vi "G#Debugger_GUI.vi"() -> ()   [LabVIEW 2020, in "G#Debugger.lvlib"]
doc: "Debugger for G# Objects."
uses:
  <vilib>/addons/_AddQ/G#Debugger/G#Debugger.lvlib
  <vilib>/addons/_AddQ/G#Object/G#Object.lvclass
  <vilib>/addons/_AddQ/G#Debugger/private/G#Debugger_DebugDialog.vi
  <vilib>/Platform/browser.llb/Open URL in Default Browser (string).vi
  <vilib>/addons/_AddQ/G#Debugger/G#Debugger_CloneUI.vi
panel:
  in  "OpClnUI":bool
  in  "RootClass":i32(ring) caption="G# Clone"
  in  "AggregatorsTags":i32(listbox)
  in  "Help":bool
  out "Application Instance":string
  in  "Window Behaviour":bool
  in  "Window Transparency":u8(slide) max=75 scale=0.0..75.0
  in  "External Create Process Running":bool
  in  "Tab Control":enum32{"Objects", "Trace", "Active Debug"}(tab)
  in  "Aggregators":i32(listbox)
  in  "AggregatesTags":i32(listbox)
  in  "Sorting":enum16{"Creation order", "By aggregation"}(ring)
  in  "Aggregates":i32(listbox)
  in  "Highlight Aggregates?":bool=TRUE
  out "To String":string
  in  "Attributes":bool
  in  "Inheritance":i32(listbox)
  in  "Destroy":bool
  in  "Object Tree":string(tree)
  in  "Refresh":bool
  out "# of Users":i32
  out "Counter":bool
  out "Ref Valid":bool
  out "Object Name":string
  out "Full Class Name":string
  in  "Poll Time (ms)":i32=200 min=0
  in  "Garbage collect":bool
  out "Object ID":u32 format="%x"
  in  "Hide Empty Classes?":bool=TRUE
  out "Owner":string
  in  "ShowAggregators":bool
  in  "Filter Expression":string
  in  "Trace Direction":bool=TRUE
  in  "Clear":bool
  in  "Save":bool
  out "Trace":string
  in  "Max Lines":u32=1000
  out "Run State":string
  out "CachedObjId":u32 caption="Object ID" format="%x"
  in  "Abort VI":bool
  in  "Run VI":bool
  in  "Open Panel":bool
  in  "DebugTree":string(tree)
  in  "Enable Active Debug":bool
  out "Icon":picture
  out "Cached Ref Valid":bool
  in  "Wait Until Done":bool=TRUE
  out "Cached Reference Class Name":string
  out "G# Version":string
  # "G# Debugger"
  # "These logs will also always appear in the NI LabVIEW Desktop Execution Trace, even without debugger running."
  # "The last created reference is automatically cashed and copied to all the new selected , opened or executed methods 'reference in'."
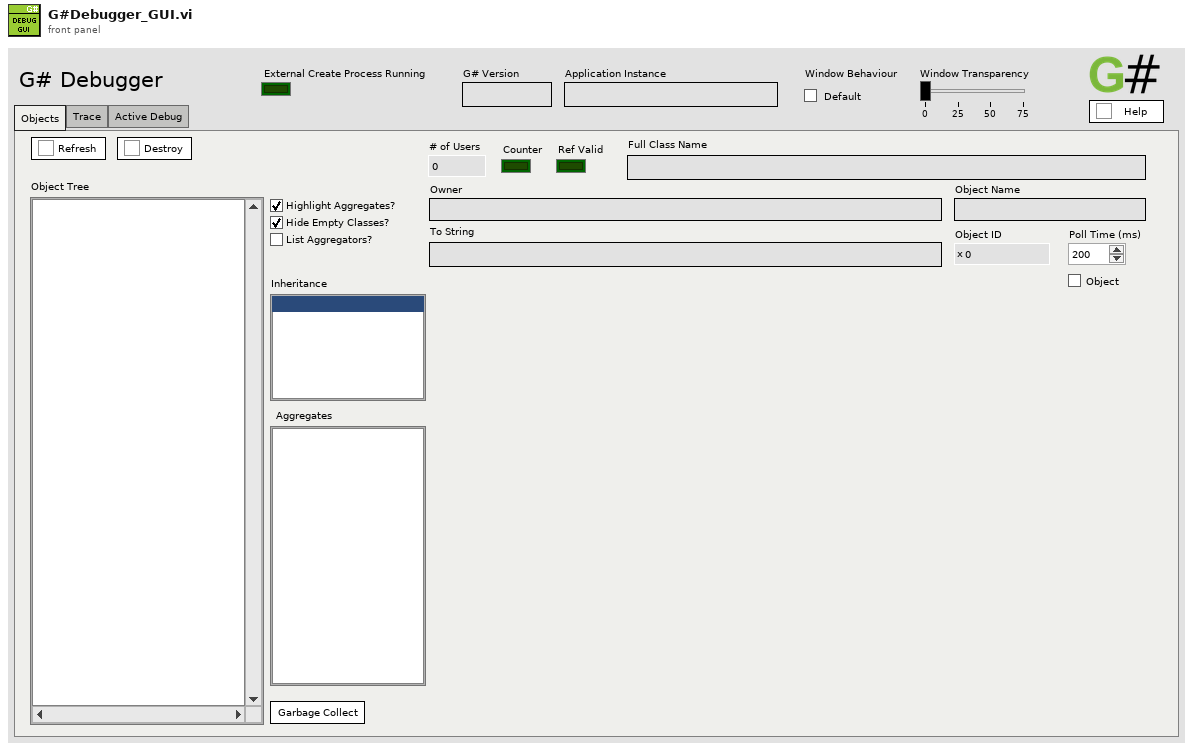
[diagram p1: front panel]
types:
  T1 = typedef "G#Debugger.lvlib/G#Debugger_Refs.ctl" = cluster{"class information dvr":refnum<data-value>, "sub panel dvr":refnum<data-value>, "GUI event":refnum<user-event>, "Active Project":refnum<vi>, "Front Panel":refnum<vi>}
  T2 = enum8{"Enabled", "Disabled", "Disabled and Grayed Out"}
  T3 = cluster{"Active Item Row Number":i32, "name":string}
  T4 = enum32{"Invalid", "Default", "Floating", "Floating/Auto-Hide", "Modal"}
  T5 = typedef "G#Debugger.lvlib/G#Debugger_SubPanelInfo.ctl" = cluster{"Ref":refnum<class "G#Object.lvclass">, "class hierarchy":T6[], "class attributes":path[], "object attributes":path[], "inheritance index":i32, "is class attributes":bool, "vi reference":refnum<vi>}
  T6 = typedef "G#Object.lvclass/G#Object_ClassHierarchy.ctl" = cluster{"ClassName":string, "FullClassName":string, "ClassPath":path, "IsLeaf":bool}
  T7 = enum32{"Bad", "Idle", "Run top level", "Running"}
  T8 = cluster{"Active Item Row Number":i32, "name":string}[]
  T9 = typedef "imagedata.ctl" = cluster{"image type":i32, "image depth":i32, "image":u8[], "mask":u8[], "colors":u32[], "Rectangle":cluster{"left":i16, "top":i16, "right":i16, "bottom":i16}}
  T10 = typedef "G#Object.lvclass/G#Object_EventType.ctl" = enum16{"Created new", "Looked up existing", "Deleted", "Forced delete", "Not deleted", "Garbage collected", "Cleared", "User", "Error", "External create object", "External create class attributes", "Created class attributes", "Run constructor", "Run constructor done", "Run open method", "Run open method done"}
  T11 = typedef "G#Object.lvclass/G#Object_ObjectInfoType.ctl" = cluster{"ObjectName":string, "ObjectID":u32, "Users":i32, "Counter":bool, "AttributeRefs":u32[], "FullClassName":string, "ClassName":string, "CreateMethod":T12, "GenericDestructorExists":bool, "Owner":string}
  T12 = typedef "G#Object.lvclass/G#Object_CreateMethod.ctl" = enum16{"Create", "Create or look up existing", "Look up existing"}
  T13 = typedef "G#Debugger.lvlib/G#Debugger_TreeElement.ctl" = cluster{"Name":string, "Tag":string, "ParentTag":string, "Position":i32}
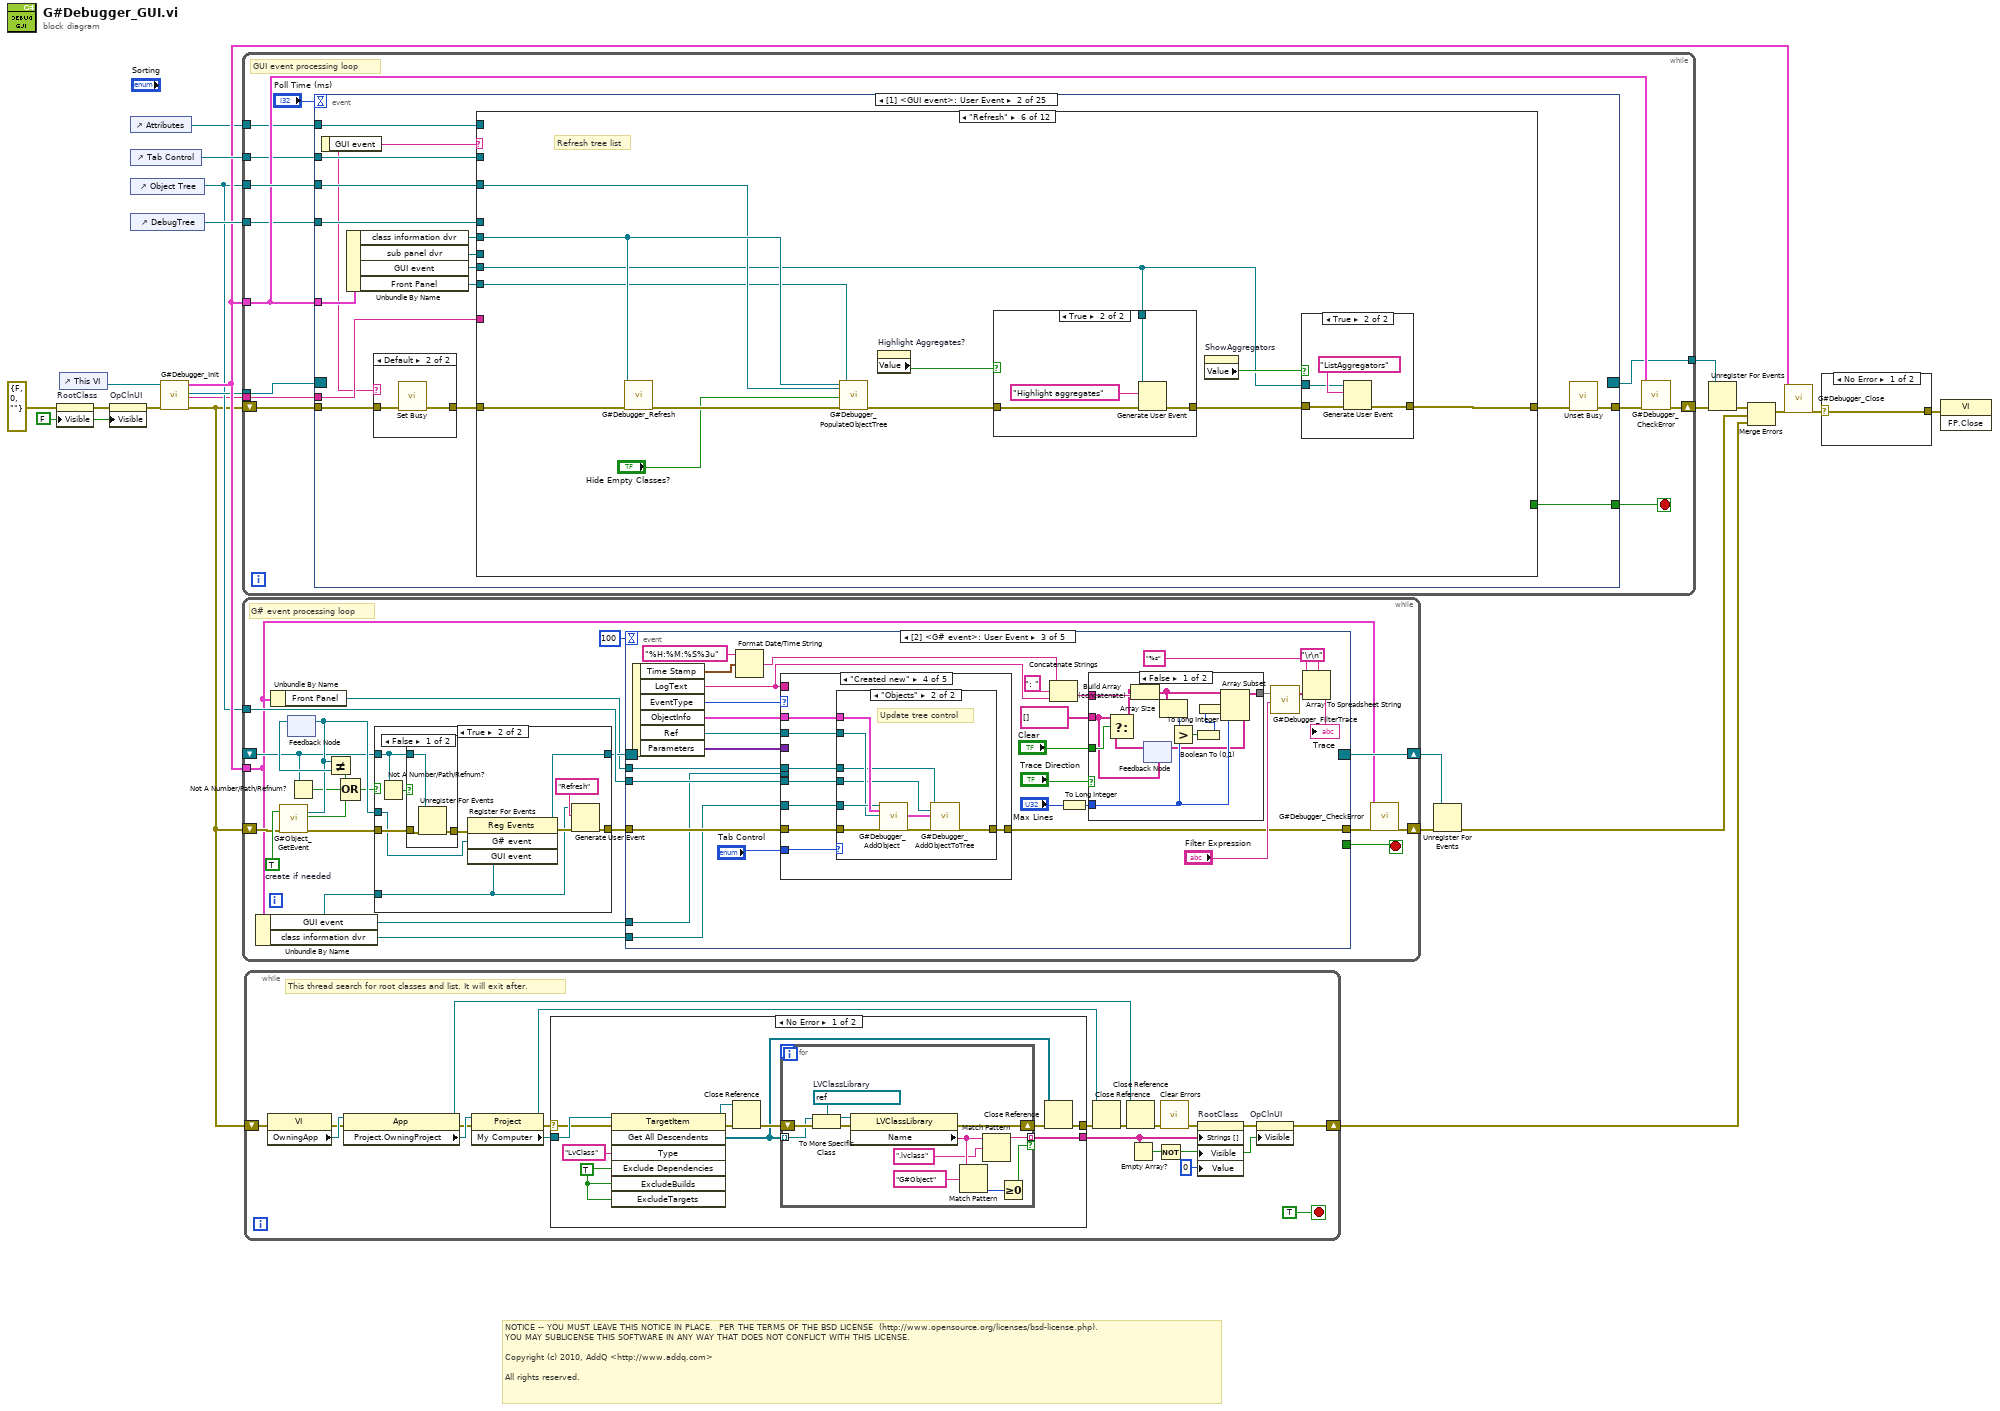
[diagram p0: block diagram]
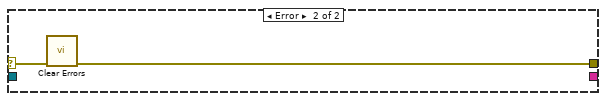
[diagram p2: hidden frame]
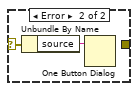
[diagram p3: hidden frame]
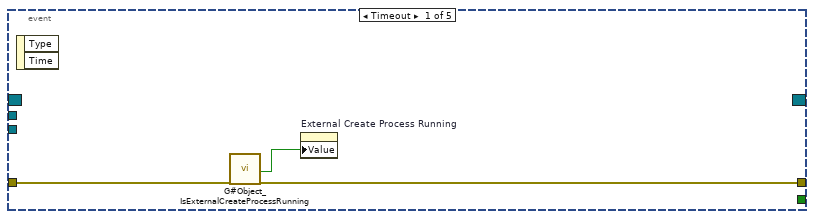
[diagram p6: hidden frame]
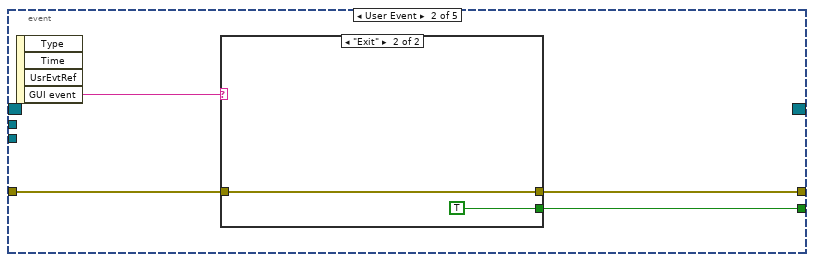
[diagram p7: hidden frame]
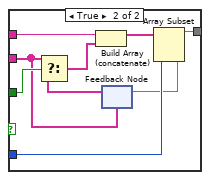
[diagram p9: hidden frame]
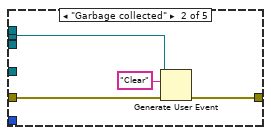
[diagram p11: hidden frame]
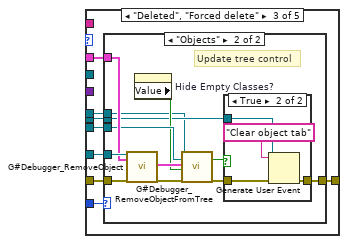
[diagram p12: hidden frame]
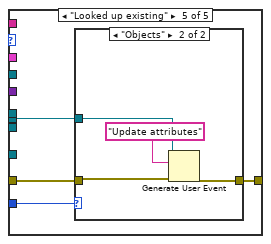
[diagram p16: hidden frame]
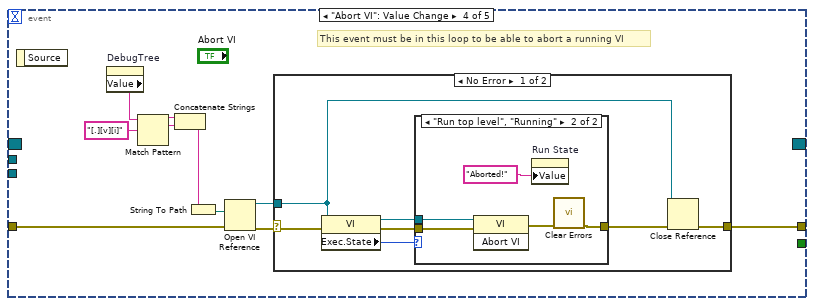
[diagram p18: hidden frame]
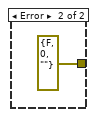
[diagram p20: hidden frame]
diagram:
  w4 = FALSE ("Visible")
  # "NOTICE -- YOU MUST LEAVE THIS NOTICE IN PLACE.  PER THE TERMS OF THE BSD LICENSE  (http://www.opensource.org/licenses/bsd-license.php).\nYOU MAY SUBLICENSE THIS SOFTWARE IN ANY WAY THAT DOES NOT CONFLICT WITH THIS LICENSE.\n\nCopyright (c) 2010, AddQ <http://www.addq.com>\n\nAll rights reserved."
  n1 = property on="RootClass" class="Ring (strict)"(error in=errorcluster {"status"=FALSE, "code"=0, "source"=""} ("error in (no error)"), "Visible"=w4) -> (error out=w3:errorcluster)  [unwired: 1 in, 1 out]
  n2 = control-ref of="This VI"() -> (w10:refnum<vi>)
  n3 = property on="OpClnUI" class="Bool"(error in=w3, "Visible"=w4) -> (error out=w1:errorcluster)  [unwired: 1 in, 1 out]
  n4 = control-ref of="Tab Control"() -> (w23:refnum<vi>)
  n5 = control-ref of="Attributes"() -> (w9:refnum<vi>)
  n6 = control-ref of="Object Tree"() -> (w12:refnum<vi>)
  n7 = control-ref of="DebugTree"() -> (w22:refnum<vi>)
  n8 = call <vilib>:"G#Debugger_Init.vi"("This VI"=w10, "error in (no error)"=w1) -> ("refs"=w21:T1, "GUI Event Registration Refnum"=w19:refnum<event-registration>, "Application Instance"=w11:string, "error out"=w6:errorcluster)  [unwired: 14 in]
  n9 = while {
    shift-right: [w34] -> w18
    shift-left: w6 -> [w29]
    tunnel: w12 -> [w36]
    tunnel: w21 -> [w32]
    tunnel: w23 -> [w31]
    tunnel: w22 -> [w30]
    tunnel: w19 -> [w28]
    tunnel: [w25] -> w17
    tunnel: w11 -> [w26]
    tunnel: w9 -> [w24]
    stop <- w35 stop-if-true
    # "GUI event processing loop"
    n10 = event shown="[1] <GUI event>: User Event" {
      selector: w28 -> [_ _ _ _ _ _ _ _ _ _ _ _ _ _ _ _ _ _ _ _ _ _ _ _ _]
      dyn-events: [_ _ _ _ _ _ _ _ _ _ _ _ _ _ _ _ _ _ _ _ _ _ _ _ _] -> w25
      timeout: "Poll Time (ms)" -> [_ _ _ _ _ _ _ _ _ _ _ _ _ _ _ _ _ _ _ _ _ _ _ _ _]
      tunnel: w29 -> [w42 w76 w473 w480 w490 w504 w508 w550 w585 w606 w613 w617 w624 w629 w632 w654 w679 w687 w727 w734 w737 w744 w759 w764 w794]
      tunnel: [w39 w78 w473 w480 w489 w503 w507 w532 w584 w605 w614 w615 w622 w626 w636 w649 w676 w686 w726 w733 w736 w744 w758 w761 w779] -> w33
      tunnel: w36 -> [_ w89 w474 w481 _ _ _ w549 _ _ w612 _ _ _ _ w648 _ _ _ _ _ _ _ w763 _]
      tunnel: [_ w88 _ _ _ FALSE _ _ _ _ _ _ _ _ _ _ _ _ _ _ _ _ _ _ _] -> w35
      tunnel: w32 -> [w46 w87 _ _ w488 w502 w506 w545 _ w604 _ w616 w623 _ w634 w645 _ w685 _ _ _ _ _ w760 _]
      tunnel: w31 -> [_ w84 _ _ _ _ _ _ _ _ _ _ _ _ _ _ _ _ _ _ _ _ _ _ _]
      tunnel: w30 -> [_ w82 _ _ _ _ _ _ _ _ _ _ _ _ _ _ _ w688 _ _ _ _ _ _ _]
      tunnel: w26 -> [_ w81 _ _ _ _ _ _ _ _ _ _ _ _ _ _ _ w684 _ _ _ _ _ _ _]
      tunnel: w24 -> [_ w74 _ _ _ _ _ _ _ _ _ _ _ _ _ _ _ _ _ _ _ _ _ _ _]
      event Timeout {
        # "redraw FP"
        n11 = event-data() -> ()  [unwired: 1 in, 2 out]
        n12 = Unbundle By Name(w46) -> ("Front Panel"=w40:refnum<vi>, "GUI event"=w45:refnum<user-event>)
        n13 = property on="Tab Control" class="TabCtl (strict)"(error in=w42) -> (error out=w43:errorcluster, "Value"=w44:enum32{"Objects", "Trace", "Active Debug"})  [unwired: 1 in, 1 out]
        n14 = case shown="Default" w44 {
          tunnel: w43 -> [w47 w57 w71]
          tunnel: w45 -> [_ w53 _]
          tunnel: [w47 w54 w70] -> w41
          frame Default {
          }
          frame "Objects" {
            # "Check for dead objects, every\n5th timeout."
            n15 = Generate User Event(user event=w53, event data cluster="Update attributes" ("event data"), error in=w57) -> (error out=w55:errorcluster)  [unwired: 1 in, 1 out]
            n16 = feedback #1(u64 0) -> (w49:u64)
            n17 = Quotient & Remainder(x=w49, y=u64 5) -> (x-y*floor(x/y)=w52:u64)  [unwired: 1 out]
            n18 = Increment(x=w49) -> (x+1=w48:u64)
            n19 = feedback-in #1(w48) -> ()
            n20 = case shown="0" w52 {
              tunnel: w55 -> [w58 w63]
              tunnel: [w58 w62] -> w54
              tunnel: w53 -> [_ w61]
              frame Default {
              }
              frame 0 {
                n21 = call <vilib>:"G#Object_CleanUp.vi"("error in (no error)"=w63) -> ("any dead objects?"=w59:bool, "error out"=w60:errorcluster)  [unwired: 17 in]
                n22 = case shown="True" w59 {
                  tunnel: w60 -> [w64 w67]
                  tunnel: [w64 w66] -> w62
                  tunnel: w61 -> [_ w65]
                  frame False {
                  }
                  frame True {
                    # "Object died, refresh"
                    n23 = Generate User Event(user event=w65, event data cluster="Refresh" ("event data"), error in=w67) -> (error out=w66:errorcluster)  [unwired: 1 in, 1 out]
                  }
                }
              }
            }
          }
          frame "Active Debug" {
            w73 = FALSE  # set
            n24 = call <vilib>:"G#Debugger_CachedObject.vi"("error in (no error)"=w71, "set"=w73) -> ("not a refnum?"=w72:bool, "error out"=w70:errorcluster)  [unwired: 15 in, 1 out]
            n25 = Not(x=w72) -> (.not. x?=w69:bool)
            n26 = property on="Cached Ref Valid" class="Bool (strict)"("Value"=w69) -> ()  [unwired: 2 in, 2 out]
          }
        }
        n27 = property class="Pnl"(reference=w40, error in=w41, "DeferPanUpdts"=FALSE ("Defer Panel Updates"), "DeferPanUpdts"=TRUE ("Defer Panel Updates")) -> (error out=w39:errorcluster)  [unwired: 1 out]
      }
      event User Event {
        n28 = event-data() -> ("GUI event"=w77:string)  [unwired: 1 in]
        n29 = Unbundle By Name(w87) -> ("class information dvr"=w86:refnum<data-value>, "sub panel dvr"=w85:refnum<data-value>, "GUI event"=w83:refnum<user-event>, "Front Panel"=w80:refnum<vi>)
        n30 = case shown="Default" w77 {
          tunnel: w76 -> [w90 w92]
          tunnel: [w90 w91] -> w75
          frame "Clear object tab", "Update attributes" {
          }
          frame Default {
            n31 = call <vilib>:"Set Busy.vi"("error in (no error)"=w92) -> ("error out"=w91:errorcluster)  [unwired: 9 in, 1 out]
          }
        }
        n32 = case shown="\"Refresh\"" w77 {
          selector: w77 -> [_ _ _ _ _ _ _ _ _ w320 _ _]
          tunnel: [w93 w94 w128 w138 w145 w151 w175 w184 w276 w316 w326 w370] -> w79
          tunnel: w75 -> [w93 w123 w129 w138 w144 w161 w179 w181 w277 w316 w331 w375]
          tunnel: [_ _ _ _ TRUE _ _ _ _ _ _ _] -> w88
          tunnel: w86 -> [_ _ _ _ _ w159 w177 w187 _ _ w329 w373]
          tunnel: w89 -> [_ w116 _ _ _ w158 w178 _ _ _ w325 w369]
          tunnel: w85 -> [_ _ _ _ _ _ _ w186 _ _ _ _]
          tunnel: w84 -> [_ w124 _ _ _ _ _ _ _ _ _ _]
          tunnel: w83 -> [_ w121 w127 _ _ w150 w174 w185 _ _ _ _]
          tunnel: w82 -> [_ w117 _ _ _ _ _ _ _ _ _ _]
          tunnel: w81 -> [_ w112 _ _ _ _ _ _ _ _ _ _]
          tunnel: w80 -> [_ w98 _ _ _ w154 w172 _ _ _ w321 w365]
          tunnel: w74 -> [_ _ _ _ _ _ _ w182 _ _ _ _]
          frame Default {
          }
          frame "Init" {
            w95 = FALSE ("ShowAggregators")
            w99 = TRUE ("Highlight Aggregates?")
            n33 = call <vilib>:"G#Object_GetRootClassVersion.vi"("error in (no error)"=w123) -> ("version"=→"G# Version":string, "error out"=w105:errorcluster)  [unwired: 17 in]
            n34 = invoke on="Method VI Panel" class="SubPanel" method="Remove VI"(error in=w105) -> (error out=w104:errorcluster)  [unwired: 2 in, 2 out]
            n35 = call <vilib>:"G#Debugger_ClearTree.vi"("Front Panel"=w98, "Tree"=w116, "error in (no error)"=w104) -> ("error out"=w114:errorcluster)  [unwired: 16 in]
            n36 = Equal?(x=w112, y="Main Application Instance") -> (x = y?=w110:bool)
            n37 = call <vilib>:"G#Object_IsExternalCreateProcessRunning.vi"("error in (no error)"=w114) -> ("external create process running?"=w106:bool, "error out"=w113:errorcluster)  [unwired: 15 in, 2 out]
            n38 = Select(t=T2."Disabled and Grayed Out" ("Disabled"), s=w110, f=T2."Enabled" ("Disabled")) -> (s? t:f=w107:T2)
            n39 = property on="External Create Process Running" class="Bool (strict)"("Value"=w106) -> ()  [unwired: 2 in, 2 out]
            n40 = property class="TabCtl (strict)"(reference=w124, error in=w113, "Value"=enum32{"Objects", "Trace", "Active Debug"}."Objects") -> (error out=w120:errorcluster)  [unwired: 1 out]
            n41 = property on="Aggregators" class="LstBox (strict)"("Visible"=FALSE) -> ()  [unwired: 2 in, 2 out]
            n42 = property on="Enable Active Debug" class="Bool (strict)"(error in=w120, "Value"=FALSE ("Enable Active Debug"), "DisabledEnum"=w107) -> (error out=w103:errorcluster)  [unwired: 1 in, 1 out]
            n43 = property on="Aggregates" class="LstBox (strict)"("Number of Rows"=u32 16) -> ()  [unwired: 2 in, 2 out]
            n44 = call <vilib>:"G#Debugger_ClearTree.vi"("Front Panel"=w98, "Tree"=w117, "error in (no error)"=w103) -> ("error out"=w115:errorcluster)  [unwired: 16 in]
            n45 = Generate User Event(user event=w121, event data cluster="Clear controls" ("event data"), error in=w115) -> (user event out=w102:refnum<user-event>, error out=w101:errorcluster)  [unwired: 1 in]
            n46 = property on="Hide Empty Classes?" class="Bool (strict)"("Value"=w99) -> ()  [unwired: 2 in, 2 out]
            n47 = property on="Highlight Aggregates?" class="Bool (strict)"("Value"=w99) -> ()  [unwired: 2 in, 2 out]
            n48 = Generate User Event(user event=w102, event data cluster="Refresh" ("event data"), error in=w101) -> (error out=w94:errorcluster)  [unwired: 1 in, 1 out]
            n49 = property on="ShowAggregators" class="Bool (strict)"("Value"=w95) -> ()  [unwired: 2 in, 2 out]
            n50 = property on="RootClass" class="Ring (strict)"("Visible"=w95) -> ()  [unwired: 2 in, 2 out]
            n51 = property on="OpClnUI" class="Bool"("Visible"=w95) -> ()  [unwired: 2 in, 2 out]
            "Application Instance" <- w112
          }
          frame "Clear controls" {
            w130 = ""
            n52 = property on="Run State" class="Str"("Value"=w130) -> ()  [unwired: 2 in, 2 out]
            n53 = property on="Cached Reference Class Name" class="Str"("Value"=w130) -> ()  [unwired: 2 in, 2 out]
            n54 = call "Empty Picture"() -> ("empty picture"=w132:picture)
            n55 = property on="Cached Ref Valid" class="Bool (strict)"("Value"=FALSE ("Counter")) -> ()  [unwired: 2 in, 2 out]
            n56 = property on="Icon" class="Pict"("Value"=w132) -> ()  [unwired: 2 in, 2 out]
            n57 = property on="Trace" class="Str"("Value"=w130) -> ()  [unwired: 2 in, 2 out]
            n58 = property on="CachedObjId" class="DigNum (strict)"("Value"=u32 0 ("Object ID")) -> ()  [unwired: 2 in, 2 out]
            n59 = Generate User Event(user event=w127, event data cluster="Clear object tab" ("event data"), error in=w129) -> (error out=w128:errorcluster)  [unwired: 1 in, 1 out]
          }
          frame "Clear object tab" {
            w134 = 0 ("Top Row")
            w135 = string[] [] ("Item Names")
            w136 = -1 ("Inheritance")
            w137 = ""
            w141 = FALSE ("Counter")
            n60 = property on="Object Name" class="Str"("Value"=w137) -> ()  [unwired: 2 in, 2 out]
            n61 = property on="To String" class="Str"("Value"=w137) -> ()  [unwired: 2 in, 2 out]
            n62 = property on="Full Class Name" class="Str"("Value"=w137) -> ()  [unwired: 2 in, 2 out]
            n63 = property on="Owner" class="Str"("Value"=w137) -> ()  [unwired: 2 in, 2 out]
            n64 = property on="Counter" class="Bool (strict)"("Value"=w141) -> ()  [unwired: 2 in, 2 out]
            n65 = property on="Ref Valid" class="Bool (strict)"("Value"=w141) -> ()  [unwired: 2 in, 2 out]
            n66 = property on="# of Users" class="DigNum (strict)"("Value"=0 ("Nr of Users")) -> ()  [unwired: 2 in, 2 out]
            n67 = property on="Object ID" class="DigNum (strict)"("Value"=u32 0 ("Object ID")) -> ()  [unwired: 2 in, 2 out]
            n68 = property on="Aggregates" class="LstBox (strict)"("Value"=w136, "Item Names"=w135, "Top Row"=w134) -> ()  [unwired: 2 in, 2 out]
            n69 = property on="Inheritance" class="LstBox (strict)"("Value"=w136, "Item Names"=w135, "Top Row"=w134) -> ()  [unwired: 2 in, 2 out]
            n70 = property on="Aggregators" class="LstBox (strict)"("Value"=w136, "Item Names"=w135, "Top Row"=w134) -> ()  [unwired: 2 in, 2 out]
          }
          frame "Exit" {
            n71 = property on="Enable Active Debug" class="Bool (strict)"(error in=w144) -> (error out=w143:errorcluster, "Value"=w142:bool)  [unwired: 1 in, 1 out]
            n72 = case shown="True" w142 {
              tunnel: [w147 w149] -> w145
              tunnel: w143 -> [w147 w148]
              frame False {
              }
              frame True {
                n73 = call <vilib>:"GarbageCollector.vi"("error in (no error)"=w148) -> ("error out"=w149:errorcluster)  [unwired: 16 in, 2 out]
              }
            }
          }
          frame "Refresh" {
            # "Refresh tree list"
            n74 = call <vilib>:"G#Debugger_Refresh.vi"("Objects dvr"=w159, "error in (no error)"=w161) -> ("error out"=w160:errorcluster)  [unwired: 17 in]
            n75 = call <vilib>:"G#Debugger_PopulateObjectTree.vi"("Objects dvr"=w159, "Tree"=w158, "hide empty classes?"="Hide Empty Classes?", "error in (no error)"=w160, "Front Panel"=w154) -> ("error out"=w156:errorcluster)  [unwired: 14 in]
            n76 = property on="Highlight Aggregates?" class="Bool (strict)"() -> ("Value"=w155:bool)  [unwired: 2 in, 2 out]
            n77 = case shown="True" w155 {
              tunnel: [w167 w170] -> w152
              tunnel: w156 -> [w167 w169]
              tunnel: w150 -> [_ w168]
              frame False {
              }
              frame True {
                n78 = Generate User Event(user event=w168, event data cluster="Highlight aggregates" ("event data"), error in=w169) -> (error out=w170:errorcluster)  [unwired: 1 in, 1 out]
              }
            }
            n79 = property on="ShowAggregators" class="Bool (strict)"() -> ("Value"=w153:bool)  [unwired: 2 in, 2 out]
            n80 = case shown="True" w153 {
              tunnel: w152 -> [w162 w165]
              tunnel: [w162 w164] -> w151
              tunnel: w150 -> [_ w163]
              frame False {
              }
              frame True {
                n81 = Generate User Event(user event=w163, event data cluster="ListAggregators" ("event data"), error in=w165) -> (error out=w164:errorcluster)  [unwired: 1 in, 1 out]
              }
            }
          }
          frame "Clear" {
            # "Clears tree and object cache"
            n82 = call <vilib>:"G#Debugger_ClearTree.vi"("Front Panel"=w172, "Tree"=w178, "error in (no error)"=w179) -> ("error out"=w180:errorcluster)  [unwired: 16 in]
            n83 = call <vilib>:"G#Debugger_Clear.vi"("Objects dvr"=w177, "error in (no error)"=w180) -> ("error out"=w176:errorcluster)  [unwired: 17 in]
            n84 = Generate User Event(user event=w174, event data cluster="Clear object tab" ("event data"), error in=w176) -> (error out=w175:errorcluster)  [unwired: 1 in, 1 out]
          }
          frame "Update attributes" {
            n85 = Empty String/Path?(string/path="Object Tree") -> (empty?=w189:bool)
            n86 = case shown="False" w189 {
              tunnel: w181 -> [w207 w261]
              tunnel: w187 -> [w206 _]
              tunnel: w186 -> [w205 w259]
              tunnel: "Object Tree" -> [w204 _]
              tunnel: "Attributes" -> [w192 _]
              tunnel: "Inheritance" -> [w203 _]
              tunnel: [w200 w255] -> w183
              tunnel: w185 -> [w195 w254]
              tunnel: w182 -> [w193 _]
              frame False {
                # "An item is selected"
                n87 = call <vilib>:"G#Debugger_UpdateAttributes.vi"("Objects dvr"=w206, "Subpanel dvr"=w205, "tag"=w204, "class attributes"=w192, "inheritance index"=w203, "error in (no error)"=w207) -> ("string"=w196:string, "Only read attributes"=w199:bool, "attributes reference"=w198:refnum<vi>, "attributes value"=w197:variant, "valid object"=w202:bool, "# of users?"=w194:i32, "error out"=w201:errorcluster)  [unwired: 7 in]
                n88 = case shown="True" w202 {
                  tunnel: w201 -> [w215 w235]
                  tunnel: [w209 w236] -> w200
                  tunnel: w199 -> [_ w225]
                  tunnel: w198 -> [_ w221]
                  tunnel: w197 -> [_ w228]
                  tunnel: w196 -> [_ w238]
                  tunnel: w195 -> [w208 _]
                  tunnel: w194 -> [_ w237]
                  tunnel: w193 -> [_ w234]
                  tunnel: w192 -> [_ w231]
                  frame False {
                    # "Subpanel info is invalid->Clear"
                    n89 = invoke on="Attributes" class="SubPanel" method="Remove VI"(error in=w215) -> (error out=w214:errorcluster)  [unwired: 2 in, 2 out]
                    n90 = call <vilib>:"G#Object_CleanUp.vi"("error in (no error)"=w214) -> ("any dead objects?"=w212:bool, "error out"=w213:errorcluster)  [unwired: 17 in]
                    n91 = case shown="True" w212 {
                      tunnel: [w217 w219] -> w210
                      tunnel: w213 -> [w217 w219]
                      tunnel: ["Clear object tab" ("event data") "Refresh" ("event data")] -> w211
                      frame False {
                      }
                      frame True {
                      }
                    }
                    n92 = Generate User Event(user event=w208, event data cluster=w211, error in=w210) -> (error out=w209:errorcluster)  [unwired: 1 in, 1 out]
                  }
                  frame True {
                    # "Valid item"
                    n93 = case shown="False" w225 {
                      tunnel: w235 -> [w251 w252]
                      tunnel: w234 -> [w248 _]
                      tunnel: [w250 w252] -> w226
                      tunnel: w221 -> [w249 _]
                      tunnel: w231 -> [w247 _]
                      frame False {
                        n94 = call <vilib>:"G#Debugger_ShowAttributes.vi"("VIRef"=w249, "SubPanel"=w248, "ClassAttributes"=w247, "error in (no error)"=w251) -> ("error out"=w250:errorcluster)  [unwired: 14 in, 1 out]
                      }
                      frame True {
                      }
                    }
                    n95 = property on="# of Users" class="DigNum (strict)"("Value"=w237) -> ()  [unwired: 2 in, 2 out]
                    n96 = Select(t="class attributes" ("y"), s=w231, f="attributes" ("y")) -> (s? t:f=w230:string)
                    n97 = Not(x=w225) -> (.not. x?=w224:bool)
                    n98 = invoke class="VI" method="Ctrl Val.Get"(reference=w221, error in=w226, "Control Name"=w230) -> (reference out=w220:refnum<vi>, error out=w227:errorcluster, "Get Control Value Variant"=w229:variant)  [unwired: 1 in, 1 out]
                    n99 = Not Equal?(x=w229, y=w228) -> (x != y?=w223:bool)
                    n100 = Or(x=w224, y=w223) -> (x .or. y?=w222:bool)
                    n101 = case shown="True" w222 {
                      tunnel: [w239 w245] -> w236
                      tunnel: w227 -> [w239 w243]
                      tunnel: w220 -> [_ w242]
                      tunnel: w230 -> [_ w241]
                      tunnel: w228 -> [_ w240]
                      frame False {
                      }
                      frame True {
                        n102 = invoke class="VI" method="Ctrl Val.Set"(reference=w242, error in=w243, "Control Name"=w241, "Value"=w240) -> (error out=w246:errorcluster)  [unwired: 1 in, 4 out]
                        n103 = property on="Attributes" class="SubPnl"(error in=w246, "DisabledEnum"=T2."Enabled" ("Disabled")) -> (error out=w245:errorcluster)  [unwired: 1 in, 1 out]
                      }
                    }
                    "To String" <- w238
                  }
                }
              }
              frame True {
                # "No item selected in tree"
                n104 = invoke on="Attributes" class="SubPanel" method="Remove VI"(error in=w261) -> (error out=w260:errorcluster)  [unwired: 2 in, 2 out]
                n105 = in-place {
                  in-place-border: w260 -> [w266]
                  in-place-border: [w264] -> w257
                  # "Force a subpanel update!"
                  n106 = in-place-dvr #2(w259) -> (w265:T5)  [unwired: 1 out]
                  n107 = Unbundle By Name(w265) -> ("vi reference"=w262:refnum<vi>)
                  n108 = Not A Number/Path/Refnum?(number/path/refnum=w262) -> (NaN/Path/Refnum?=w263:bool)
                  n109 = case shown="False" w263 {
                    tunnel: w266 -> [w269 w270]
                    tunnel: [w268 w270] -> w264
                    tunnel: w262 -> [w267 _]
                    frame False {
                      n110 = Close Reference(reference=w267, error in (no error)=w269) -> (error out=w268:errorcluster)
                    }
                    frame True {
                    }
                  }
                  n111 = in-place-dvr #2(w265) -> (w258:errorcluster)  [unwired: 1 out]
                }
                n112 = Merge Errors(w258, w257) -> (w256:errorcluster)
                n113 = Generate User Event(user event=w254, event data cluster="Clear object tab" ("event data"), error in=w256) -> (error out=w255:errorcluster)  [unwired: 1 in, 1 out]
              }
            }
            n114 = call <vilib>:"Clear Errors.vi"("error in (no error)"=w183) -> ("error out"=w184:errorcluster)  [unwired: 5 in, 1 out]
          }
          frame "Run VI" {
            n115 = property on="DebugTree" class="Tree (strict)"() -> ("Value"=w271:string)  [unwired: 2 in, 2 out]
            n116 = Match Pattern(string=w271, regular expression="[.][v][i]") -> (before substring=w274:string, match substring=w273:string)  [unwired: 1 in, 2 out]
            n117 = Concatenate Strings(w274, w273) -> (w272:string)
            n118 = String To Path(string=w272) -> (path=w278:path)
            n119 = Open VI Reference(vi path=w278, error in (no error)=w277) -> (vi reference=w280:refnum<vi>, error out=w279:errorcluster)  [unwired: 4 in]
            n120 = case shown="No Error" w279 {
              selector: w279 -> [w285 _]
              tunnel: [w291 errorcluster {"status"=FALSE, "code"=0, "source"=""} ("error in (no error)")] -> w276
              tunnel: w280 -> [w284 _]
              tunnel: w278 -> [w289 _]
              frame No Error {
                n121 = stacked-sequence {
                  tunnel: w289 -> [w297]
                  tunnel: [w297] -> w288
                  frame #0 {
                    "Run State" <- "Running..." ("Run State")
                  }
                }
                n122 = property class="VI"(reference=w284, error in=w285) -> (error out=w282:errorcluster, "Exec.State"=w283:T7, "Exec.IsReentrant"=w286:bool)  [unwired: 1 out]
                n123 = case shown="Default" w283 {
                  tunnel: [FALSE TRUE w294 w295] -> w287
                  tunnel: w286 -> [_ _ w294 w295]
                  frame Default {
                  }
                  frame "Idle" {
                  }
                  frame "Run top level" {
                  }
                  frame "Running" {
                  }
                }
                n124 = case shown="True" w287 {
                  tunnel: [w303 w311] -> w290
                  tunnel: w282 -> [w303 w306]
                  tunnel: w288 -> [w302 _]
                  tunnel: [w299 w314] -> w281
                  tunnel: w283 -> [w298 _]
                  tunnel: w284 -> [_ w307]
                  frame False {
                    n125 = Strip Path(path=w302) -> (name=w301:string)  [unwired: 1 out]
                    n126 = Format Into String(format string="%s is not reentrant or in idle execution state! (%s)", w301, w298) -> (resulting string=w299:string)  [unwired: 2 in, 1 out]
                  }
                  frame True {
                    n127 = call <vilib>:"G#Debugger_RunVI.vi"("vi reference"=w307, "wait until done"="Wait Until Done", "error in (no error)"=w306) -> ("class name"=→"Cached Reference Class Name":string, "object ID"=→"CachedObjId":u32, "message"=w310:string, "not a refnum?"=w305:bool, "error out"=w311:errorcluster)  [unwired: 12 in]
                    n128 = Not(x=w305) -> (.not. x?=→"Cached Ref Valid":bool)
                    n129 = Select(t=w310, s="Wait Until Done", f="Run state is not available!") -> (s? t:f=w314:string)
                  }
                }
                n130 = Close Reference(reference=w284, error in (no error)=w290) -> (error out=w291:errorcluster)
                n131 = property on="Run State" class="Str"("Value"=w281) -> ()  [unwired: 2 in, 2 out]
              }
              frame Error {
              }
            }
          }
          frame "Wait".."Wb" {
            n132 = Decimal String To Number(string=w320, offset=5, default (0L)=u32 0 ("default (0 I32)")) -> (number=w317:u32)  [unwired: 1 out]
            n133 = Wait (ms)(milliseconds to wait=w317) -> ()  [unwired: 1 out]
          }
          frame "Highlight aggregates" {
            n134 = property on="Property Node" class="Tree (strict)"(reference=w325, error in=w331) -> (error out=w330:errorcluster, "Value"=w328:string)  [unwired: 1 out]
            n135 = call <vilib>:"G#Debugger_GetObjectFromTag.vi"("Objects dvr"=w329, "Tag"=w328, "class attributes"=FALSE, "error in (no error)"=w330) -> ("Ref"=w324:refnum<class "G#Object.lvclass">, "Found"=w322:bool, "error out"=w323:errorcluster)  [unwired: 13 in]
            n136 = case shown="True" w322 {
              tunnel: [w332 w340] -> w326
              tunnel: w325 -> [_ w352]
              tunnel: w324 -> [_ w351]
              tunnel: w323 -> [w332 w349]
              tunnel: w321 -> [_ w339]
              frame False {
              }
              frame True {
                w346 = TRUE  # remove duplicates
                # "redraw FP"
                n137 = property on="Attributes" class="Bool (strict)"(error in=w349) -> (error out=w348:errorcluster, "Value"=w347:bool)  [unwired: 1 in, 1 out]
                n138 = call <vilib>:"G#Object_GetAggregatedObjects.vi"("reference in"=w351, "class attributes (F)"=w347, "remove duplicates (F)"=w346, "error in (no error)"=w348) -> ("aggregated objects"=w345:refnum<class "G#Object.lvclass">[], "error out"=w344:errorcluster)  [unwired: 12 in, 2 out]
                n139 = for {
                  tunnel: w345 -> [w355] mode=indexing
                  shift-right: [w356] -> w350
                  shift-left: w344 -> [w358]
                  tunnel: [w357] -> w333 mode=indexing if=w353
                  n140 = call-dynamic "NotARefNum.vi"("reference in"=w355) -> ("not a refnum?"=w354:bool)  [unwired: 1 in, 1 out]
                  n141 = case shown="False" w354 {
                    tunnel: w355 -> [w363 _]
                    tunnel: w358 -> [w362 w364]
                    tunnel: [w360 _] -> w357
                    tunnel: [w359 w364] -> w356
                    frame False {
                      # "ObjectIDs are the\ntags in the object tree"
                      n142 = call-dynamic "GetObjectID.vi"("reference in"=w363, "error in (no error)"=w362) -> ("object ID"=w361:u32, "error out"=w359:errorcluster)  [unwired: 15 in, 1 out]
                      n143 = Number To Decimal String(number=w361) -> (decimal integer string=w360:string)  [unwired: 1 in]
                    }
                    frame True {
                    }
                  }
                  n144 = Not(x=w354) -> (.not. x?=w353:bool)
                }
                n145 = control-ref of="Aggregates"() -> (w338:refnum<vi>)
                n146 = control-ref of="AggregatesTags"() -> (w337:refnum<vi>)
                n147 = Array Size(array=w333) -> (size(s)=w336:i32)
                n148 = call <vilib>:"G#Debugger_Highlight.vi"("Tree"=w352, "Aggregates"=w338, "ObjectIDs"=w333, "error in (no error)"=w350, "AggregatesTags"=w337) -> ("error out"=w341:errorcluster)  [unwired: 14 in]
                n149 = Greater Or Equal?(x=w336, y=8) -> (x >= y?=w335:bool)
                n150 = property class="Pnl"(reference=w339, error in=w341, "DeferPanUpdts"=FALSE ("Defer Panel Updates"), "DeferPanUpdts"=TRUE ("Defer Panel Updates")) -> (error out=w340:errorcluster)  [unwired: 1 out]
                n151 = property on="Aggregates" class="LstBox (strict)"("Scrollbar Visible"=w335) -> ()  [unwired: 2 in, 2 out]
              }
            }
          }
          frame "ListAggregators" {
            n152 = property on="Property Node" class="Tree (strict)"(reference=w369, error in=w375) -> (error out=w374:errorcluster, "Value"=w372:string)  [unwired: 1 out]
            n153 = call <vilib>:"G#Debugger_GetObjectFromTag.vi"("Objects dvr"=w373, "Tag"=w372, "class attributes"=FALSE, "error in (no error)"=w374) -> ("Ref"=w368:refnum<class "G#Object.lvclass">, "Found"=w366:bool, "error out"=w367:errorcluster)  [unwired: 13 in]
            n154 = case shown="True" w366 {
              tunnel: [w376 w396] -> w370
              tunnel: w369 -> [_ _]
              tunnel: w368 -> [_ w395]
              tunnel: w367 -> [w376 w401]
              tunnel: w365 -> [_ w381]
              frame False {
              }
              frame True {
                # "redraw FP"
                n155 = call-dynamic "GetObjectID.vi"("reference in"=w395) -> ("object ID"=w378:u32)  [unwired: 16 in, 2 out]
                n156 = property on="Attributes" class="Bool (strict)"(error in=w401) -> (error out=w400:errorcluster, "Value"=w399:bool)  [unwired: 1 in, 1 out]
                n157 = Equal To 0?(x=w378) -> (x = 0?=w377:bool)
                n158 = case shown="False" w377 {
                  tunnel: w400 -> [w413 w464]
                  tunnel: w399 -> [w412 _]
                  tunnel: w378 -> [w406 _]
                  tunnel: [w405 w464] -> w394
                  tunnel: [w403 _] -> w387
                  tunnel: [w402 _] -> w385
                  frame False {
                    w411 = TRUE  # remove duplicates
                    n159 = call <vilib>:"G#Object_GetAllObjects.vi"("only refs (F)"=TRUE) -> ("all refs"=w408:refnum<class "G#Object.lvclass">[])  [unwired: 15 in, 3 out]
                    n160 = for {
                      tunnel: w412 -> [w420]
                      tunnel: w411 -> [w419]
                      tunnel: [w417] -> w410 mode=indexing if=w414
                      shift-right: [w418] -> w409
                      shift-left: w413 -> [w421]
                      tunnel: w408 -> [w416] mode=indexing
                      tunnel: [w416] -> w404 mode=indexing if=w414
                      n161 = call-dynamic "NotARefNum.vi"("reference in"=w416) -> ("not a refnum?"=w415:bool)  [unwired: 1 in, 1 out]
                      n162 = Not(x=w415) -> (.not. x?=w414:bool)
                      n163 = case shown="False" w415 {
                        tunnel: w421 -> [w428 w433]
                        tunnel: w420 -> [w427 _]
                        tunnel: w419 -> [w426 _]
                        tunnel: [w425 w433] -> w418
                        tunnel: w416 -> [w424 _]
                        tunnel: [w422 _] -> w417
                        frame False {
                          n164 = call <vilib>:"G#Object_GetAggregatedObjects.vi"("reference in"=w424, "class attributes (F)"=w427, "remove duplicates (F)"=w426, "error in (no error)"=w428) -> ("aggregated objects"=w423:refnum<class "G#Object.lvclass">[], "error out"=w425:errorcluster)  [unwired: 12 in, 2 out]
                          n165 = for {
                            tunnel: w423 -> [w432] mode=indexing
                            tunnel: [w431] -> w422 mode=indexing if=w429
                            n166 = call-dynamic "NotARefNum.vi"("reference in"=w432) -> ("not a refnum?"=w430:bool, "reference out"=w431:refnum<class "G#Object.lvclass">)  [unwired: 1 in]
                            n167 = Not(x=w430) -> (.not. x?=w429:bool)
                          }
                        }
                        frame True {
                        }
                      }
                    }
                    n168 = for {
                      tunnel: w410 -> [w444] mode=indexing
                      shift-right: [w440] -> w405
                      shift-left: w409 -> [w443]
                      tunnel: [w436] -> w403 mode=indexing if=w434
                      tunnel: w406 -> [w442]
                      tunnel: w404 -> [w439] mode=indexing
                      tunnel: [w435] -> w402 mode=indexing if=w434
                      # "ObjectIDs are the\ntags in the object tree"
                      n169 = for {
                        tunnel: w444 -> [w455] mode=indexing
                        tunnel: w442 -> [w453]
                        tunnel: [w450] -> w434
                        shift-right: [w451] -> w441
                        shift-left: w443 -> [w454]
                        stop <- w450 stop-if-true
                        n170 = call-dynamic "GetObjectID.vi"("reference in"=w455, "error in (no error)"=w454) -> ("object ID"=w452:u32, "error out"=w451:errorcluster)  [unwired: 15 in, 1 out]
                        n171 = Equal?(x=w453, y=w452) -> (x = y?=w450:bool)
                      }
                      n172 = case shown="True" w434 {
                        tunnel: w441 -> [w456 w463]
                        tunnel: [w456 w462] -> w440
                        tunnel: w439 -> [_ w458]
                        tunnel: [_ w460] -> w438
                        tunnel: [_ w459] -> w437
                        tunnel: [_ w457] -> w435
                        frame False {
                        }
                        frame True {
                          n173 = call-dynamic "GetObjectID.vi"("reference in"=w458) -> ("object ID"=w457:u32)  [unwired: 16 in, 2 out]
                          n174 = call-dynamic "GetObjectStatus.vi"("reference in"=w458, "simple info (F)"=TRUE, "error in (no error)"=w463) -> ("class name"=w460:string, "object name"=w459:string, "error out"=w462:errorcluster)  [unwired: 5 in, 9 out]
                        }
                      }
                      n175 = disable-structure shown="Enabled" {
                        disable-tunnel: w438 -> [w448 _]
                        disable-tunnel: w437 -> [w447 w449]
                        disable-tunnel: [w445 w449] -> w436
                        frame Enabled {
                          n176 = Format Into String(format string="%s:%s", w448, w447) -> (resulting string=w445:string)  [unwired: 2 in, 1 out]
                        }
                        frame Disabled {
                        }
                      }
                    }
                  }
                  frame True {
                  }
                }
                n177 = for {
                  tunnel: w385 -> [w469] mode=indexing
                  tunnel: w387 -> [w470] mode=indexing
                  tunnel: [w468] -> w389 mode=indexing
                  n178 = Bundle(cluster=T3 {"Active Item Row Number"=0, "name"=""}, "Active Item Row Number"=w469, "name"=w470) -> (w468:T3)
                }
                n179 = Sort 1D Array(array=w385) -> (sorted array=w384:u32[])
                n180 = Array Size(array=w384) -> (size(s)=w392:i32)
                n181 = Greater Or Equal?(x=w392, y=7) -> (x >= y?=w391:bool)
                n182 = Number To Decimal String(number=w384) -> (decimal integer string=w382:string[])  [unwired: 1 in]
                n183 = property on="Aggregators" class="LstBox (strict)"("Scrollbar Visible"=w391) -> ()  [unwired: 2 in, 2 out]
                n184 = Sort 1D Array(array=w389) -> (sorted array=w388:T8)
                n185 = for {
                  tunnel: w388 -> [w466] mode=indexing
                  tunnel: [w465] -> w386 mode=indexing
                  n186 = Unbundle By Name(w466) -> ("name"=w465:string)
                }
                n187 = property on="Aggregators" class="LstBox (strict)"(error in=w394, "Item Names"=w386) -> (error out=w393:errorcluster)  [unwired: 1 in, 1 out]
                n188 = control-ref of="AggregatorsTags"() -> (w390:refnum<vi>)
                n189 = property on="Property Node" class="LstBox (strict)"(reference=w390, "Item Names"=w382, "Value"=-1, "Top Row"=0) -> ()  [unwired: 1 in, 2 out]
                n190 = property class="Pnl"(reference=w381, error in=w393, "DeferPanUpdts"=FALSE ("Defer Panel Updates"), "DeferPanUpdts"=TRUE ("Defer Panel Updates")) -> (error out=w396:errorcluster)  [unwired: 1 out]
              }
            }
          }
        }
        n191 = call <vilib>:"Unset Busy.vi"("error in (no error)"=w79) -> ("error out"=w78:errorcluster)  [unwired: 10 in]
      }
      event "Aggregates": Double Click {
        n192 = event-data() -> ()  [unwired: 1 in, 1 out]
        n193 = control-ref of="AggregatesTags"() -> (w472:refnum<vi>)
        n194 = control-ref of="Aggregates"() -> (w471:refnum<vi>)
        n195 = property class="LstBox (strict)"(reference=w472) -> ("Item Names"=w476:string[])  [unwired: 1 in, 2 out]
        n196 = property class="LstBox (strict)"(reference=w471) -> ("Value"=w477:i32)  [unwired: 1 in, 2 out]
        n197 = Index Array(array=w476, index=w477) -> (element=w475:string)
        n198 = property class="Tree (strict)"(reference=w474, "Val(Sgnl)"=w475) -> ()  [unwired: 1 in, 2 out]
      }
      event "Aggregators": Double Click {
        n199 = event-data() -> ()  [unwired: 1 in, 1 out]
        n200 = control-ref of="AggregatorsTags"() -> (w479:refnum<vi>)
        n201 = control-ref of="Aggregators"() -> (w478:refnum<vi>)
        n202 = property class="LstBox (strict)"(reference=w478) -> ("Value"=w484:i32)  [unwired: 1 in, 2 out]
        n203 = property class="LstBox (strict)"(reference=w479) -> ("Item Names"=w483:string[])  [unwired: 1 in, 2 out]
        n204 = Index Array(array=w483, index=w484) -> (element=w482:string)
        n205 = property class="Tree (strict)"(reference=w481, "Val(Sgnl)"=w482) -> ()  [unwired: 1 in, 2 out]
      }
      event "ShowAggregators": Value Change {
        n206 = event-data() -> ("NewVal"=w486:bool)  [unwired: 1 in]
        n207 = Unbundle By Name(w488) -> ("GUI event"=w487:refnum<user-event>)
        n208 = property on="Aggregators" class="LstBox (strict)"("Visible"=w486) -> ()  [unwired: 2 in, 2 out]
        n209 = case shown="True" w486 {
          tunnel: w490 -> [w492 w496]
          tunnel: [w492 w495] -> w489
          tunnel: w487 -> [_ w494]
          tunnel: [u32 16 ("Number of Rows") u32 7 ("Number of Rows")] -> w485
          frame False {
          }
          frame True {
            n210 = Generate User Event(user event=w494, event data cluster="ListAggregators" ("event data"), error in=w496) -> (error out=w495:errorcluster)  [unwired: 1 in, 1 out]
          }
        }
        n211 = property on="Aggregates" class="LstBox (strict)"("Number of Rows"=w485) -> ()  [unwired: 2 in, 2 out]
      }
      event Panel Close? {
        n212 = event-data() -> ()  [unwired: 1 in, 3 out]
        n213 = Unbundle By Name(w502) -> ("GUI event"=w499:refnum<user-event>)
        n214 = Generate User Event(user event=w499, event data cluster="Exit" ("event data"), error in=w504) -> (error out=w503:errorcluster)  [unwired: 1 in, 1 out]
        n215 = event-data("Discard?"=TRUE) -> ()  [unwired: 1 in, 1 out]
      }
      event "Tab Control": Value Change {
        n216 = event-data() -> ("NewVal"=w509:enum32{"Objects", "Trace", "Active Debug"})  [unwired: 1 in, 4 out]
        n217 = Unbundle By Name(w506) -> ("GUI event"=w505:refnum<user-event>)
        n218 = case shown="\"Objects\"" w509 {
          tunnel: w508 -> [w513 w516]
          tunnel: [w515 w516] -> w507
          tunnel: w505 -> [w511 _]
          frame "Objects" {
            # "Refresh tree control"
            n219 = Generate User Event(user event=w511, event data cluster="Clear object tab" ("event data"), error in=w513) -> (error out=w512:errorcluster)  [unwired: 1 in, 1 out]
            n220 = Generate User Event(user event=w511, event data cluster="Refresh" ("event data"), error in=w512) -> (error out=w515:errorcluster)  [unwired: 1 in, 1 out]
          }
          frame Default {
          }
        }
      }
      event "Object Tree": Value Change {
        w561 = TRUE  # simple info
        n221 = event-data() -> ()  [unwired: 1 in, 1 out]
        n222 = property class="Tree (strict)"(reference=w549, error in=w550) -> (error out=w531:errorcluster, "Value"=w548:string)  [unwired: 1 out]
        n223 = Unbundle By Name(w545) -> ("class information dvr"=w544:refnum<data-value>, "GUI event"=w526:refnum<user-event>)
        n224 = property on="Attributes" class="Bool (strict)"(error in=w531) -> (error out=w530:errorcluster, "Value"=w529:bool)  [unwired: 1 in, 1 out]
        n225 = call <vilib>:"G#Debugger_GetObjectFromTag.vi"("Objects dvr"=w544, "Tag"=w548, "class attributes"=w529, "error in (no error)"=w530) -> ("Ref"=w555:refnum<class "G#Object.lvclass">, "error out"=w562:errorcluster)  [unwired: 13 in, 1 out]
        n226 = call-dynamic "GetObjectStatus.vi"("reference in"=w555, "simple info (F)"=w561, "error in (no error)"=w562) -> ("full class name"=→"Full Class Name":string, "# of users?"=→"# of Users":i32, "class name"=w533:string, "reference out"=w553:refnum<class "G#Object.lvclass">, "not a refnum?"=w558:bool, "object name"=→"Object Name":string, "counter?"=→"Counter":bool, "error out"=w554:errorcluster)  [unwired: 5 in, 4 out]
        n227 = Not(x=w558) -> (.not. x?=→"Ref Valid":bool)
        n228 = property on="Cached Reference Class Name" class="Str"("Value"=w533) -> ()  [unwired: 2 in, 2 out]
        n229 = call <vilib>:"G#Object_GetClassHierarchy.vi"("reference in"=w553, "error in (no error)"=w554) -> ("reference out"=w542:refnum<class "G#Object.lvclass">, "class hierarchy"=w552:T6[], "error out"=w543:errorcluster)  [unwired: 15 in]
        n230 = call-dynamic "GetObjectID.vi"("reference in"=w542, "error in (no error)"=w543) -> ("reference out"=w538:refnum<class "G#Object.lvclass">, "object ID"=w534:u32, "error out"=w539:errorcluster)  [unwired: 15 in]
        "Object ID" <- w534
        n231 = property on="CachedObjId" class="DigNum (strict)"("Value"=w534) -> ()  [unwired: 2 in, 2 out]
        n232 = for {
          tunnel: w552 -> [w574] mode=indexing
          tunnel: [w573] -> w547 mode=indexing
          n233 = Unbundle By Name(w574) -> ("ClassName"=w573:string)
        }
        n234 = call-dynamic "G#Object_GetOwner.vi"("reference in"=w538, "error in (no error)"=w539) -> ("reference out"=w536:refnum<class "G#Object.lvclass">, "owner"=→"Owner":string, "error out"=w537:errorcluster)  [unwired: 15 in]
        n235 = call <vilib>:"G#Debugger_CachedObject.vi"("cached object"=w536, "error in (no error)"=w537, "set"=TRUE) -> ("error out"=w528:errorcluster)  [unwired: 14 in, 2 out]
        n236 = case shown="True" "Highlight Aggregates?" {
          tunnel: w528 -> [w568 w572]
          tunnel: [w568 w571] -> w527
          tunnel: w526 -> [_ w569]
          frame False {
          }
          frame True {
            n237 = Generate User Event(user event=w569, event data cluster="Highlight aggregates" ("event data"), error in=w572) -> (error out=w571:errorcluster)  [unwired: 1 in, 1 out]
          }
        }
        n238 = Array Size(array=w547) -> (size(s)=w518:i32)
        n239 = Decrement(x=w518) -> (x-1=w546:i32)
        n240 = property on="Inheritance" class="LstBox (strict)"("Item Names"=w547, "Value"=w546, "Top Row"=0) -> ()  [unwired: 2 in, 2 out]
        n241 = Generate User Event(user event=w526, event data cluster="Update attributes" ("event data"), error in=w527) -> (user event out=w522:refnum<user-event>, error out=w524:errorcluster)  [unwired: 1 in]
        n242 = Greater Or Equal?(x=w518, y=8) -> (x >= y?=w520:bool)
        n243 = case shown="True" "ShowAggregators" {
          tunnel: w524 -> [w563 w566]
          tunnel: [w563 w565] -> w523
          tunnel: w522 -> [_ w564]
          frame False {
          }
          frame True {
            n244 = Generate User Event(user event=w564, event data cluster="ListAggregators" ("event data"), error in=w566) -> (error out=w565:errorcluster)  [unwired: 1 in, 1 out]
          }
        }
        n245 = property on="Inheritance" class="LstBox (strict)"("Scrollbar Visible"=w520) -> ()  [unwired: 2 in, 2 out]
        n246 = call <vilib>:"Clear Errors.vi"("error in (no error)"=w523) -> ("error out"=w532:errorcluster)  [unwired: 5 in, 1 out]
      }
      event "DebugTree": Value Change {
        n247 = event-data() -> ("NewVal"=w579:string)  [unwired: 1 in, 4 out]
        n248 = Match Pattern(string=w579, regular expression="[.][v][i]") -> (before substring=w577:string, match substring=w576:string)  [unwired: 1 in, 2 out]
        n249 = Concatenate Strings(w577, w576) -> (w575:string)
        n250 = String To Path(string=w575) -> (path=w580:path)
        n251 = Open VI Reference(vi path=w580, error in (no error)=w585) -> (vi reference=w583:refnum<vi>, error out=w582:errorcluster)  [unwired: 4 in]
        n252 = case shown="No Error" w582 {
          selector: w582 -> [w589 _]
          tunnel: [w592 w602] -> w584
          tunnel: w583 -> [w587 _]
          tunnel: [w590 w603] -> w581
          frame No Error {
            n253 = call <vilib>:"G#Debugger_SetCachedRef.vi"("MethodVIref"=w587, "error in (no error)"=w589) -> ("error out"=w588:errorcluster)  [unwired: 17 in]
            n254 = invoke on="Method VI Panel" class="SubPanel" method="Insert VI"(error in=w588, "VI Ref"=w587) -> (error out=w586:errorcluster)  [unwired: 2 in, 3 out]
            n255 = case shown="No Error" w586 {
              selector: w586 -> [w596 _]
              tunnel: [w595 w598] -> w591
              tunnel: w587 -> [w597 _]
              tunnel: [w593 w600] -> w590
              frame No Error {
                n256 = invoke class="VI" method="VI Icon.Get as Image Data"(reference=w597, error in=w596) -> (error out=w595:errorcluster, "ImageData"=w594:T9)  [unwired: 4 in, 4 out]
                n257 = call <vilib>:"Draw Flattened Pixmap.vi"("image data"=w594) -> ("new picture"=w593:picture)  [unwired: 8 in]
              }
              frame Error {
                n258 = vi-ref "G#Debugger.lvlib:G#Debugger_DebugDialog.vi"() -> (w599:refnum<vi>)
                n259 = invoke on="Method VI Panel" class="SubPanel" method="Insert VI"("VI Ref"=w599) -> (error out=w598:errorcluster)  [unwired: 3 in, 3 out]
                n260 = call "Empty Picture"() -> ("empty picture"=w600:picture)
              }
            }
            n261 = Close Reference(reference=w587, error in (no error)=w591) -> (error out=w592:errorcluster)
          }
          frame Error {
            n262 = invoke on="Method VI Panel" class="SubPanel" method="Remove VI"(error in=errorcluster {"status"=FALSE, "code"=0, "source"=""} ("error in (no error)")) -> (error out=w602:errorcluster)  [unwired: 2 in, 2 out]
            n263 = call "Empty Picture"() -> ("empty picture"=w603:picture)
          }
        }
        "Icon" <- w581
      }
      event "Run VI": Value Change {
        # "We need to fire a new event so we don't lock up the UI event."
        n264 = event-data() -> ()  [unwired: 1 in, 5 out]
        n265 = Unbundle By Name(w604) -> ("GUI event"=w607:refnum<user-event>)
        n266 = Generate User Event(user event=w607, event data cluster="Run VI" ("event data"), error in=w606) -> (error out=w605:errorcluster)  [unwired: 1 in, 1 out]
      }
      event "Attributes": Value Change {
        n267 = event-data() -> ()  [unwired: 1 in, 5 out]
        n268 = property class="Tree (strict)"(reference=w612, error in=w613) -> (reference out=w610:refnum<vi>, error out=w611:errorcluster, "Value"=w609:string)
        n269 = property class="Tree (strict)"(reference=w610, error in=w611, "Val(Sgnl)"=w609) -> (error out=w614:errorcluster)  [unwired: 1 out]
      }
      event "Inheritance": Value Change {
        n270 = event-data() -> ()  [unwired: 1 in, 5 out]
        n271 = Unbundle By Name(w616) -> ("GUI event"=w618:refnum<user-event>)
        n272 = Generate User Event(user event=w618, event data cluster="Update attributes" ("event data"), error in=w617) -> (error out=w615:errorcluster)  [unwired: 1 in, 1 out]
      }
      event "Refresh", "Hide Empty Classes?": Value Change {
        n273 = event-data() -> ()  [unwired: 1 in, 5 out]
        n274 = Unbundle By Name(w623) -> ("GUI event"=w620:refnum<user-event>)
        n275 = Generate User Event(user event=w620, event data cluster="Refresh" ("event data"), error in=w624) -> (error out=w622:errorcluster)  [unwired: 1 in, 1 out]
      }
      event "Clear": Value Change {
        n276 = event-data() -> ()  [unwired: 1 in, 5 out]
        n277 = call <vilib>:"G#Object_SendUserEvent.vi"("text"="Debugger clearing display!" ("Text"), "error in (no error)"=w629) -> ("error out"=w627:errorcluster)  [unwired: 16 in, 1 out]
        n278 = property on="Trace" class="Str"(error in=w627, "Value"="") -> (error out=w626:errorcluster)  [unwired: 1 in, 1 out]
      }
      event "Garbage collect": Value Change {
        n279 = event-data() -> ()  [unwired: 1 in, 5 out]
        n280 = Unbundle By Name(w634) -> ("GUI event"=w633:refnum<user-event>)
        n281 = call <vilib>:"G#Object_SendUserEvent.vi"("text"="Debugger garbage collected!" ("Text"), "error in (no error)"=w632) -> ("error out"=w640:errorcluster)  [unwired: 16 in, 1 out]
        n282 = call <vilib>:"GarbageCollector.vi"("only from same owner as caller? (T)"=FALSE, "error in (no error)"=w640) -> ("error out"=w631:errorcluster)  [unwired: 15 in, 2 out]
        n283 = call <vilib>:"Clear Errors.vi"("error in (no error)"=w631) -> ("error out"=w630:errorcluster)  [unwired: 5 in, 1 out]
        n284 = property on="Enable Active Debug" class="Bool (strict)"() -> ("Value"=w639:bool)  [unwired: 2 in, 2 out]
        n285 = case shown="True" w639 {
          tunnel: w630 -> [w642 w644]
          tunnel: [w642 w643] -> w635
          frame False {
          }
          frame True {
            n286 = call <vilib>:"G#Object_StartExternalCreateProcess.vi"("error in (no error)"=w644) -> ("error out"=w643:errorcluster)  [unwired: 18 in]
          }
        }
        n287 = property on="External Create Process Running" class="Bool (strict)"("Value"=w639) -> ()  [unwired: 2 in, 2 out]
        n288 = Generate User Event(user event=w633, event data cluster="Clear" ("event data"), error in=w635) -> (error out=w636:errorcluster)  [unwired: 1 in, 1 out]
      }
      event "Destroy": Value Change {
        n289 = event-data() -> ()  [unwired: 1 in, 5 out]
        n290 = Unbundle By Name(w645) -> ("class information dvr"=w646:refnum<data-value>)
        n291 = property class="Tree (strict)"(reference=w648, error in=w654) -> (error out=w653:errorcluster, "Value"=w647:string)  [unwired: 1 out]
        n292 = call <vilib>:"G#Debugger_GetObjectFromTag.vi"("Objects dvr"=w646, "Tag"=w647, "error in (no error)"=w653) -> ("Ref"=w650:refnum<class "G#Object.lvclass">, "Found"=w651:bool, "error out"=w652:errorcluster)  [unwired: 14 in]
        n293 = case shown="True" w651 {
          tunnel: w652 -> [w655 w661]
          tunnel: w650 -> [_ w663]
          tunnel: [w655 w662] -> w649
          tunnel: w648 -> [_ w660]
          tunnel: w647 -> [_ w659]
          frame False {
          }
          frame True {
            w665 = TRUE  # Simple Info
            n294 = call <vilib>:"G#Debugger_NavigateToPreviousTreeItem.vi"("Tree"=w660, "Tag"=w659, "error in (no error)"=w661) -> ("error out"=w658:errorcluster)  [unwired: 16 in]
            n295 = call <vilib>:"G#Object_SendUserEvent.vi"("text"="Debugger killed object!" ("Text"), "error in (no error)"=w658) -> ("error out"=w657:errorcluster)  [unwired: 16 in, 1 out]
            n296 = call-dynamic "GetObjectStatus.vi"("reference in"=w663, "simple info (F)"=w665, "error in (no error)"=w657) -> ("# of users?"=w664:i32, "error out"=w666:errorcluster)  [unwired: 5 in, 10 out]
            n297 = for {
              N: w664 -> [_]
              tunnel: [w667] -> w662
              tunnel: w666 -> [w670]
              tunnel: w663 -> [w669]
              # "Loop users"
              n298 = call-dynamic "NotARefNum.vi"("reference in"=w669) -> ("not a refnum?"=w668:bool)  [unwired: 1 in, 1 out]
              n299 = case shown="False" w668 {
                tunnel: [w672 w675] -> w667
                tunnel: w670 -> [w674 w675]
                tunnel: w669 -> [w673 _]
                frame False {
                  n300 = call-dynamic "Destroy.vi"("reference in"=w673, "error in (no error)"=w674) -> ("error out"=w671:errorcluster)  [unwired: 16 in, 1 out]
                  n301 = call <vilib>:"Clear Errors.vi"("error in (no error)"=w671) -> ("error out"=w672:errorcluster)  [unwired: 5 in, 1 out]
                }
                frame True {
                }
              }
            }
          }
        }
      }
      event "Save": Value Change {
        n302 = event-data() -> ()  [unwired: 1 in, 5 out]
        n303 = property on="Trace" class="Str"() -> ("Value"=w678:string)  [unwired: 2 in, 2 out]
        n304 = Write to Text File(text=w678, error in=w679) -> (error out=w677:errorcluster)  [unwired: 2 in, 2 out]
        n305 = call <vilib>:"Clear Errors.vi"("error in (no error)"=w677) -> ("error out"=w676:errorcluster)  [unwired: 5 in, 1 out]
      }
      event "Enable Active Debug": Value Change {
        n306 = event-data() -> ("NewVal"=w680:bool)  [unwired: 1 in, 4 out]
        n307 = Select(t="Debugger enabled active debug!" ("Text"), s=w680, f="Debugger disabled active debug!" ("Text")) -> (s? t:f=w691:string)
        n308 = call <vilib>:"G#Object_SendUserEvent.vi"("text"=w691, "error in (no error)"=w687) -> ("error out"=w683:errorcluster)  [unwired: 16 in, 1 out]
        n309 = call <vilib>:"G#Object_EnableDebug.vi"("set (F)"=TRUE, "debug enable (F)"=w680, "error in (no error)"=w683) -> ("error out"=w682:errorcluster)  [unwired: 14 in, 2 out]
        n310 = case shown="False" w680 {
          tunnel: w682 -> [w702 w710]
          tunnel: [w704 w712] -> w686
          tunnel: w688 -> [w703 w711]
          tunnel: w685 -> [w693 w709]
          tunnel: w684 -> [_ w706]
          frame False {
            n311 = Unbundle By Name(w693) -> ("Front Panel"=w692:refnum<vi>)
            n312 = property on="Cached Reference Class Name" class="Str"("Value"="") -> ()  [unwired: 2 in, 2 out]
            n313 = call <vilib>:"G#Debugger_CachedObject.vi"("cached object"=refnum<class "G#Object.lvclass"> refnum, "error in (no error)"=w702, "set"=TRUE) -> ("error out"=w701:errorcluster)  [unwired: 14 in, 2 out]
            n314 = call <vilib>:"GarbageCollector.vi"("error in (no error)"=w701) -> ("error out"=w695:errorcluster)  [unwired: 16 in, 2 out]
            n315 = property on="CachedObjId" class="DigNum (strict)"("Value"=u32 0 ("CachedObjId")) -> ()  [unwired: 2 in, 2 out]
            n316 = call "Empty Picture"() -> ("empty picture"=w696:picture)
            n317 = invoke on="Method VI Panel" class="SubPanel" method="Remove VI"(error in=w695) -> (error out=w694:errorcluster)  [unwired: 2 in, 2 out]
            n318 = property on="Icon" class="Pict"("Value"=w696) -> ()  [unwired: 2 in, 2 out]
            n319 = call <vilib>:"G#Debugger_ClearTree.vi"("Front Panel"=w692, "Tree"=w703, "error in (no error)"=w694) -> ("error out"=w704:errorcluster)  [unwired: 16 in]
          }
          frame True {
            n320 = Unbundle By Name(w709) -> ("Front Panel"=w705:refnum<vi>, "Active Project"=w708:refnum<vi>)
            n321 = Not A Number/Path/Refnum?(number/path/refnum=w708) -> (NaN/Path/Refnum?=w707:bool)
            n322 = case shown="False" w707 {
              tunnel: [w718 w723] -> w712
              tunnel: w711 -> [w717 _]
              tunnel: w710 -> [w715 w723]
              tunnel: w708 -> [w714 _]
              tunnel: w706 -> [_ w722]
              tunnel: w705 -> [w713 _]
              frame False {
                n323 = call <vilib>:"G#Object_StartExternalCreateProcess.vi"("error in (no error)"=w715) -> ("error out"=w716:errorcluster)  [unwired: 18 in]
                n324 = call <vilib>:"G#Debugger_PopulateActiveDebugTree.vi"("Front Panel"=w713, "Tree"=w717, "Active Project"=w714, "error in (no error)"=w716) -> ("error out"=w718:errorcluster)  [unwired: 15 in]
              }
              frame True {
                n325 = Format Into String(format string="%s not valid anymore!", w722) -> (resulting string=w721:string)  [unwired: 2 in, 1 out]
                n326 = property on="Enable Active Debug" class="Bool (strict)"("Value"=FALSE ("Enable Active Debug")) -> ()  [unwired: 2 in, 2 out]
                n327 = One Button Dialog(message=w721) -> ()  [unwired: 1 in, 1 out]
              }
            }
          }
        }
      }
      event "Window Transparency": Value Change {
        n328 = event-data() -> ()  [unwired: 1 in, 5 out]
        n329 = control-ref of="This VI"() -> (w728:refnum<vi>)
        n330 = Not Equal To 0?(x="Window Transparency") -> (x != 0?=w724:bool)
        n331 = property class="VI"(reference=w728, error in=w727, "FP:Transparency"="Window Transparency", "FP:RunTransparently"=w724) -> (error out=w726:errorcluster)  [unwired: 1 out]
      }
      event "Window Behaviour": Value Change {
        n332 = event-data() -> ()  [unwired: 1 in, 5 out]
        n333 = Select(t=T4."Floating" ("Front Panel Window:Behavior"), s="Window Behaviour", f=T4."Default" ("Front Panel Window:Behavior")) -> (s? t:f=w729:T4)
        n334 = property class="VI"(error in=w734, "FP.Behavior"=w729) -> (error out=w733:errorcluster)  [unwired: 1 in, 1 out]
      }
      event "External Create Process Running": Value Change {
        n335 = event-data() -> ()  [unwired: 1 in, 5 out]
        n336 = case shown="False" "External Create Process Running" {
          tunnel: w737 -> [w739 w741]
          tunnel: [w738 w740] -> w736
          frame False {
            n337 = call <vilib>:"G#Object_StopExternalCreateProcess.vi"("error in (no error)"=w739) -> ("error out"=w738:errorcluster)  [unwired: 17 in, 1 out]
          }
          frame True {
            n338 = call <vilib>:"G#Object_StartExternalCreateProcess.vi"("error in (no error)"=w741) -> ("error out"=w740:errorcluster)  [unwired: 18 in]
          }
        }
      }
      event "Help": Value Change {
        n339 = event-data() -> ()  [unwired: 1 in, 5 out]
        n340 = property class="App"() -> ("OS.Name"=w742:string, "OS.Version"=w743:string)  [unwired: 2 in, 2 out]
        n341 = case shown="\"Windows\"..\"Windowt\"" w742 {
          tunnel: w743 -> [_ _]
          frame Default {
            n342 = call-poly <vilib>:"Open URL in Default Browser.vi"("URL"="http://www.addq.se/document/GsharpOnlineManual.htm" ("message")) -> ()  [unwired: 5 in, 2 out]
          }
          frame "Windows".."Windowt" {
            w753 = TRUE  # run minimized? (F)
            w754 = FALSE  # wait until completion? (T)
            n343 = VI Library() -> (path=w752:path)
            n344 = Strip Path(path=w752) -> (stripped path=w751:path)  [unwired: 1 out]
            n345 = Build Path(base path=w751, name or relative path="help") -> (appended path=w749:path)
            n346 = Build Path(base path=w749, name or relative path="_AddQ") -> (appended path=w747:path)
            n347 = call <vilib>:"System Exec.vi"("run minimized? (F)"=w753, "wait until completion? (T)"=w754, "working directory"=w747, "command line"="cmd /c hh.exe \"Gsharp.chm::GsharpDebugger.htm\"") -> ()  [unwired: 4 in, 4 out]
          }
        }
      }
      event "Filter Expression": Value Change {
        n348 = event-data() -> ("NewVal"=w756:string)  [unwired: 1 in, 4 out]
        n349 = Format Into String(format string="Changed filter expression to '%s'!" ("text"), w756) -> (resulting string=w755:string)  [unwired: 2 in, 1 out]
        n350 = call <vilib>:"G#Object_SendUserEvent.vi"("text"=w755, "error in (no error)"=w759) -> ("error out"=w758:errorcluster)  [unwired: 16 in, 1 out]
      }
      event "Highlight Aggregates?": Value Change {
        n351 = event-data() -> ("NewVal"=w762:bool)  [unwired: 1 in, 4 out]
        n352 = case shown="False" w762 {
          tunnel: w764 -> [w772 w775]
          tunnel: w763 -> [w771 _]
          tunnel: [w767 w776] -> w761
          tunnel: w760 -> [w766 w774]
          frame False {
            # "redraw FP"
            n353 = call <vilib>:"G#Debugger_Highlight.vi"("Tree"=w771, "error in (no error)"=w772) -> ("error out"=w768:errorcluster)  [unwired: 17 in]
            n354 = Unbundle By Name(w766) -> ("Front Panel"=w765:refnum<vi>)
            n355 = property class="Pnl"(reference=w765, error in=w768, "DeferPanUpdts"=FALSE ("Defer Panel Updates"), "DeferPanUpdts"=TRUE ("Defer Panel Updates")) -> (error out=w767:errorcluster)  [unwired: 1 out]
          }
          frame True {
            n356 = Unbundle By Name(w774) -> ("GUI event"=w773:refnum<user-event>)
            n357 = Generate User Event(user event=w773, event data cluster="Highlight aggregates" ("event data"), error in=w775) -> (error out=w776:errorcluster)  [unwired: 1 in, 1 out]
          }
        }
      }
      event "OpClnUI": Value Change {
        n358 = event-data() -> ()  [unwired: 1 in, 1 out]
        n359 = property on="RootClass" class="Ring (strict)"(error in=w794) -> (error out=w782:errorcluster, "Strings []"=w793:string[], "Value"=w792:i32)  [unwired: 1 in, 1 out]
        n360 = Index Array(array=w793, index=w792) -> (element=w786:string)
        n361 = vi-ref "G#Debugger.lvlib:G#Debugger_CloneUI.vi"() -> (w790:refnum<vi>)
        n362 = property class="VI"(reference=w790, error in=w782) -> (reference out=w785:refnum<vi>, error out=w780:errorcluster, "Path"=w789:path)
        n363 = Open VI Reference(type specifier VI Refnum (for type only)=refnum<vi> refnum, vi path=w789, options=128, error in (no error)=w780) -> (vi reference=w787:refnum<vi>, error out=w791:errorcluster)  [unwired: 2 in]
        n364 = call-by-ref "Start Asynchronous Call"(reference=w787, error in=w791, "RootClass"=w786) -> (reference out=w784:refnum<vi>, error out=w783:errorcluster)  [unwired: 19 in]
        n365 = Close Reference(reference=w784, error in (no error)=w783) -> (error out=w781:errorcluster)
        n366 = Close Reference(reference=w785, error in (no error)=w781) -> (error out=w779:errorcluster)
      }
    }
    n367 = call <vilib>:"G#Debugger_CheckError.vi"("refs"=w32, "error in (no error)"=w33) -> ("error out"=w34:errorcluster)  [unwired: 17 in]
  }
  n368 = while {
    shift-right: [w816] -> w15
    shift-left: w6 -> [w802]
    tunnel: w21 -> [w796]
    shift-right: [w813] -> w13
    shift-left: _ -> [w801]
    tunnel: w12 -> [w812]
    stop <- w814 stop-if-true
    w803 = TRUE  # create if needed
    # "G# event processing loop"
    n369 = Unbundle By Name(w796) -> ("GUI event"=w798:refnum<user-event>, "class information dvr"=w797:refnum<data-value>)
    n370 = Unbundle By Name(w796) -> ("Front Panel"=w795:refnum<vi>)
    n371 = call <vilib>:"G#Object_GetEvent.vi"("create if needed (T)"=w803, "error in (no error)"=w802) -> ("G# event"=w809:refnum<user-event>, "created new"=w808:bool, "error out"=w804:errorcluster)  [unwired: 13 in, 2 out]
    n372 = feedback #3() -> (w810:refnum<user-event>)  [unwired: 1 in]
    n373 = feedback-in #3(w809) -> ()
    n374 = Not A Number/Path/Refnum?(number/path/refnum=w801) -> (NaN/Path/Refnum?=w805:bool)
    n375 = Not Equal?(x=w809, y=w810) -> (x != y?=w807:bool)
    n376 = Compound Arithmetic op=OR(w807, w805, w808) -> (w806:bool)
    n377 = case shown="True" w806 {
      tunnel: w804 -> [w818 w828]
      tunnel: w801 -> [w817 w826]
      tunnel: [w818 w822] -> w799
      tunnel: w809 -> [_ w824]
      tunnel: [w817 w823] -> w800
      tunnel: w798 -> [_ w819]
      frame False {
      }
      frame True {
        n378 = Not A Number/Path/Refnum?(number/path/refnum=w826) -> (NaN/Path/Refnum?=w827:bool)
        n379 = case shown="False" w827 {
          tunnel: w828 -> [w830 w832]
          tunnel: [w831 w832] -> w825
          tunnel: w826 -> [w829 _]
          frame False {
            n380 = Unregister For Events(event registration refnum=w829, error in=w830) -> (error out=w831:errorcluster)
          }
          frame True {
          }
        }
        n381 = register-events(error in=w825, w824, w819) -> (reference out=w823:refnum<event-registration>, error out=w820:errorcluster)  [unwired: 1 in]
        n382 = Generate User Event(user event=w819, event data cluster="Refresh" ("event data"), error in=w820) -> (error out=w822:errorcluster)  [unwired: 1 in, 1 out]
      }
    }
    n383 = event shown="[2] <G# event>: User Event" {
      selector: w800 -> [_ _ _ _ _]
      dyn-events: [_ _ _ _ _] -> w813
      timeout: 100 -> [_ _ _ _ _]
      tunnel: w799 -> [w834 w838 w869 w958 w979]
      tunnel: [w833 w837 w847 w956 w978] -> w815
      tunnel: [_ w836 _ _ _] -> w814
      tunnel: w812 -> [_ _ w867 _ _]
      tunnel: w798 -> [_ _ w845 _ _]
      tunnel: w797 -> [_ _ w844 _ _]
      tunnel: w795 -> [_ _ w843 _ _]
      event Timeout {
        n384 = event-data() -> ()  [unwired: 1 in, 2 out]
        n385 = call <vilib>:"G#Object_IsExternalCreateProcessRunning.vi"("error in (no error)"=w834) -> ("external create process running?"=w835:bool, "error out"=w833:errorcluster)  [unwired: 15 in, 2 out]
        n386 = property on="External Create Process Running" class="Bool (strict)"("Value"=w835) -> ()  [unwired: 2 in, 2 out]
      }
      event User Event {
        n387 = event-data() -> ("GUI event"=w839:string)  [unwired: 1 in, 3 out]
        n388 = case shown="\"Exit\"" w839 {
          tunnel: w838 -> [w840 w842]
          tunnel: [w840 w842] -> w837
          tunnel: [_ TRUE] -> w836
          frame Default {
          }
          frame "Exit" {
          }
        }
      }
      event User Event {
        n389 = event-data() -> ("Time Stamp"=w863:timestamp, "LogText"=w860:string, "EventType"=w870:T10, "ObjectInfo"=w868:T11, "Ref"=w861:refnum<class "G#Object.lvclass">, "Parameters"=w859:variant[])  [unwired: 1 in]
        n390 = Format Date/Time String(time format string (%c)="%H:%M:%S%3u", seconds (now)=w863) -> (date/time string=w862:string)  [unwired: 1 in]
        n391 = case shown="\"Created new\"" w870 {
          tunnel: w869 -> [w891 w892 w903 w929 w942]
          tunnel: [w891 w894 w899 w924 w941] -> w847
          tunnel: w868 -> [_ _ w901 w928 _]
          tunnel: w845 -> [_ w893 w897 _ w940]
          tunnel: w844 -> [_ _ w902 w927 _]
          tunnel: w867 -> [_ _ w900 w926 _]
          tunnel: "Tab Control" -> [_ _ w898 w925 w943]
          tunnel: w861 -> [_ _ _ w923 _]
          tunnel: w860 -> [_ _ _ _ _]
          tunnel: w859 -> [_ _ _ _ _]
          tunnel: w843 -> [_ _ w896 w922 _]
          frame Default {
          }
          frame "Garbage collected" {
            n392 = Generate User Event(user event=w893, event data cluster="Clear" ("event data"), error in=w892) -> (error out=w894:errorcluster)  [unwired: 1 in, 1 out]
          }
          frame "Deleted", "Forced delete" {
            n393 = case shown="\"Objects\"" w898 {
              tunnel: w903 -> [w904 w914]
              tunnel: w902 -> [_ w913]
              tunnel: w901 -> [_ w912]
              tunnel: w900 -> [_ w911]
              tunnel: [w904 w907] -> w899
              tunnel: w897 -> [_ w906]
              tunnel: w896 -> [_ w905]
              frame Default {
              }
              frame "Objects" {
                # "Update tree control"
                n394 = call <vilib>:"G#Debugger_RemoveObject.vi"("Objects dvr"=w913, "ObjectInfo"=w912, "error in (no error)"=w914) -> ("Elements"=w916:T13, "error out"=w915:errorcluster)  [unwired: 15 in]
                n395 = property on="Hide Empty Classes?" class="Bool (strict)"() -> ("Value"=w910:bool)  [unwired: 2 in, 2 out]
                n396 = call <vilib>:"G#Debugger_RemoveObjectFromTree.vi"("Front Panel"=w905, "Tree"=w911, "TreeElement"=w916, "hide empty classes?"=w910, "error in (no error)"=w915) -> ("EmptyTree?"=w908:bool, "error out"=w909:errorcluster)  [unwired: 13 in]
                n397 = case shown="True" w908 {
                  tunnel: w909 -> [w917 w920]
                  tunnel: [w917 w921] -> w907
                  tunnel: w906 -> [_ w919]
                  frame False {
                  }
                  frame True {
                    n398 = Generate User Event(user event=w919, event data cluster="Clear object tab" ("event data"), error in=w920) -> (error out=w921:errorcluster)  [unwired: 1 in, 1 out]
                  }
                }
              }
            }
          }
          frame "Created new" {
            n399 = case shown="\"Objects\"" w925 {
              tunnel: w929 -> [w930 w939]
              tunnel: [w930 w938] -> w924
              tunnel: w928 -> [_ w937]
              tunnel: w927 -> [_ w936]
              tunnel: w926 -> [_ w934]
              tunnel: w923 -> [_ w935]
              tunnel: w922 -> [_ w931]
              frame Default {
              }
              frame "Objects" {
                # "Update tree control"
                n400 = call <vilib>:"G#Debugger_AddObject.vi"("Objects dvr"=w936, "ObjectInfo"=w937, "Ref"=w935, "error in (no error)"=w939) -> ("Elements"=w933:T13[], "error out"=w932:errorcluster)  [unwired: 14 in]
                n401 = call <vilib>:"G#Debugger_AddObjectToTree.vi"("Front Panel"=w931, "Tree"=w934, "Elements"=w933, "error in (no error)"=w932) -> ("error out"=w938:errorcluster)  [unwired: 15 in]
              }
            }
          }
          frame "Looked up existing" {
            n402 = case shown="\"Objects\"" w943 {
              tunnel: w942 -> [w944 w946]
              tunnel: [w944 w947] -> w941
              tunnel: w940 -> [_ w945]
              frame Default {
              }
              frame "Objects" {
                n403 = Generate User Event(user event=w945, event data cluster="Update attributes" ("event data"), error in=w946) -> (error out=w947:errorcluster)  [unwired: 1 in, 1 out]
              }
            }
          }
        }
        n404 = Concatenate Strings(w862, ": " ("string"), w860) -> (w854:string)
        n405 = To Long Integer(number="Max Lines") -> (32bit integer=w846:i32)
        n406 = case shown="False" "Trace Direction" {
          tunnel: w846 -> [w879 w890]
          tunnel: w854 -> [w876 w887]
          tunnel: [w875 w888] -> w850
          tunnel: "Clear" -> [w874 w886]
          tunnel: string[] [] -> [w871 w883]
          frame False {
            n407 = feedback #4(w871) -> (w873:string[])
            n408 = Select(t=w871, s=w874, f=w873) -> (s? t:f=w872:string[])
            n409 = Build Array (concatenate)(w872, w876) -> (w877:string[])
            n410 = Array Size(array=w877) -> (size(s)=w882:i32)
            n411 = Greater?(x=w882, y=w879) -> (0:w881:bool)
            n412 = Boolean To (0,1)(Boolean=w881) -> (0, 1=w880:i16)
            n413 = To Long Integer(number=w880) -> (32bit integer=w878:i32)
            n414 = Array Subset(array=w877, index=w878, length=w879) -> (w875:string[])
            n415 = feedback-in #4(w875) -> ()
          }
          frame True {
            n416 = feedback #5(w883) -> (w885:string[])
            n417 = Select(t=w883, s=w886, f=w885) -> (s? t:f=w884:string[])
            n418 = Build Array (concatenate)(w887, w884) -> (w889:string[])
            n419 = Array Subset(array=w889, length=w890) -> (w888:string[])  [unwired: 1 in]
            n420 = feedback-in #5(w888) -> ()
          }
        }
        n421 = call <vilib>:"G#Debugger_FilterTrace.vi"("TraceIn"=w850, "FilterExpression"="Filter Expression") -> ("TraceOut"=w849:string[])  [unwired: 17 in]
        n422 = Array To Spreadsheet String(delimiter (Tab)="\r\n", array=w849, 3:"%s" ("format string")) -> (spreadsheet string=→"Trace":string)
      }
      event "Abort VI": Value Change {
        # "This event must be in this loop to be able to abort a running VI"
        n423 = event-data() -> ()  [unwired: 1 in, 1 out]
        n424 = property on="DebugTree" class="Tree (strict)"() -> ("Value"=w949:string)  [unwired: 2 in, 2 out]
        n425 = Match Pattern(string=w949, regular expression="[.][v][i]") -> (before substring=w952:string, match substring=w951:string)  [unwired: 1 in, 2 out]
        n426 = Concatenate Strings(w952, w951) -> (w950:string)
        n427 = String To Path(string=w950) -> (path=w957:path)
        n428 = Open VI Reference(vi path=w957, error in (no error)=w958) -> (vi reference=w955:refnum<vi>, error out=w954:errorcluster)  [unwired: 4 in]
        n429 = case shown="No Error" w954 {
          selector: w954 -> [w959 _]
          tunnel: [w962 errorcluster {"status"=FALSE, "code"=0, "source"=""} ("error out")] -> w956
          tunnel: w955 -> [w960 _]
          frame No Error {
            n430 = property class="VI"(reference=w960, error in=w959) -> (reference out=w963:refnum<vi>, error out=w964:errorcluster, "Exec.State"=w965:T7)
            n431 = case shown="\"Run top level\", \"Running\"" w965 {
              tunnel: w964 -> [w966 w971]
              tunnel: w963 -> [_ w970]
              tunnel: [w966 w968] -> w961
              frame "Bad", Default {
              }
              frame "Run top level", "Running" {
                n432 = invoke class="VI" method="Abort VI"(reference=w970, error in=w971) -> (error out=w969:errorcluster)  [unwired: 1 in, 2 out]
                n433 = property on="Run State" class="Str"("Value"="Aborted!") -> ()  [unwired: 2 in, 2 out]
                n434 = call <vilib>:"Clear Errors.vi"("error in (no error)"=w969) -> ("error out"=w968:errorcluster)  [unwired: 5 in, 1 out]
              }
            }
            n435 = Close Reference(reference=w960, error in (no error)=w961) -> (error out=w962:errorcluster)
          }
          frame Error {
          }
        }
      }
      event "Open Panel": Value Change; "DebugTree": Double Click {
        # "This event must be in this loop to be able to open a running VI"
        n436 = event-data() -> ()  [unwired: 1 in, 4 out]
        n437 = Match Pattern(string="DebugTree", regular expression="[.][v][i]") -> (before substring=w975:string, match substring=w973:string)  [unwired: 1 in, 2 out]
        n438 = Concatenate Strings(w975, w973) -> (w974:string)
        n439 = String To Path(string=w974) -> (path=w982:path)
        n440 = Open VI Reference(vi path=w982, error in (no error)=w979) -> (vi reference=w980:refnum<vi>, error out=w981:errorcluster)  [unwired: 4 in]
        n441 = case shown="No Error" w981 {
          selector: w981 -> [w984 _]
          tunnel: [w988 errorcluster {"status"=FALSE, "code"=0, "source"=""} ("error in (no error)")] -> w978
          tunnel: w980 -> [w985 _]
          frame No Error {
            n442 = invoke on="Method VI Panel" class="SubPanel" method="Remove VI"(error in=w984) -> (error out=w983:errorcluster)  [unwired: 2 in, 2 out]
            n443 = call <vilib>:"G#Debugger_SetCachedRef.vi"("MethodVIref"=w985, "error in (no error)"=w983) -> ("error out"=w986:errorcluster)  [unwired: 17 in]
            n444 = case shown="No Error" w986 {
              selector: w986 -> [w991 _]
              tunnel: [w994 errorcluster {"status"=FALSE, "code"=0, "source"=""} ("error out")] -> w987
              tunnel: w985 -> [w993 _]
              frame No Error {
                n445 = vi-ref "G#Debugger.lvlib:G#Debugger_DebugDialog.vi"() -> (w989:refnum<vi>)
                n446 = invoke on="Method VI Panel" class="SubPanel" method="Insert VI"(error in=w991, "VI Ref"=w989) -> (error out=w990:errorcluster)  [unwired: 2 in, 3 out]
                n447 = call "Empty Picture"() -> ("empty picture"=w992:picture)
                n448 = property on="Icon" class="Pict"("Value"=w992) -> ()  [unwired: 2 in, 2 out]
                n449 = property class="VI"(reference=w993, error in=w990, "Front Panel.Open"=TRUE ("Front Panel Window:Open")) -> (error out=w994:errorcluster)  [unwired: 1 out]
              }
              frame Error {
              }
            }
            n450 = Close Reference(reference=w985, error in (no error)=w987) -> (error out=w988:errorcluster)
          }
          frame Error {
          }
        }
      }
    }
    n451 = call <vilib>:"G#Debugger_CheckError.vi"("refs"=w796, "error in (no error)"=w815) -> ("error out"=w816:errorcluster)  [unwired: 17 in]
  }
  n452 = while {
    shift-right: [w999] -> w5
    shift-left: w6 -> [w1000]
    stop <- TRUE stop-if-true
    # "This thread search for root classes and list. It will exit after."
    n453 = property class="VI"(error in=w1000) -> (error out=w1014:errorcluster, "OwningApp"=w1015:refnum<vi>)  [unwired: 1 in, 1 out]
    n454 = property class="App"(reference=w1015, error in=w1014) -> (reference out=w1013:refnum<vi>, error out=w1007:errorcluster, "Project.OwningProject"=w1008:refnum<vi>)
    n455 = property class="Project"(reference=w1008, error in=w1007) -> (reference out=w1012:refnum<vi>, error out=w1010:errorcluster, "My Computer"=w1011:refnum<vi>)
    n456 = case shown="No Error" w1010 {
      selector: w1010 -> [w1022 w1042]
      tunnel: w1011 -> [w1026 _]
      tunnel: [w1019 w1041] -> w1009
      tunnel: [w1018 _] -> w1017
      frame No Error {
        w1027 = TRUE ("ExcludeDependencies")
        n457 = invoke class="TargetItem" method="Get All Descendents"(reference=w1026, error in=w1022, "Type"="LvClass", "Exclude Dependencies"=w1027, "ExcludeBuilds"=w1027, "ExcludeTargets"=w1027) -> (reference out=w1025:refnum<vi>, error out=w1023:errorcluster, "All Descendents"=w1021:refnum<vi>[])  [unwired: 1 in, 4 out]
        n458 = Close Reference(reference=w1025, error in (no error)=w1023) -> (error out=w1024:errorcluster)
        n459 = for {
          tunnel: w1021 -> [w1039] mode=indexing
          shift-right: [w1029] -> w1020
          shift-left: w1024 -> [w1040]
          tunnel: [w1031] -> w1018 mode=indexing if=w1030
          w1038 = refnum<vi> refnum  # LVClassLibrary
          n460 = To More Specific Class(target class=w1038, reference=w1039, error in=w1040) -> (specific class reference=w1032:refnum<vi>, error out=w1033:errorcluster)
          n461 = property class="LVClassLibrary"(reference=w1032, error in=w1033) -> (error out=w1029:errorcluster, "Name"=w1036:string)  [unwired: 1 out]
          n462 = Match Pattern(string=w1036, regular expression="G#Object" ("string")) -> (offset past match=w1037:i32)  [unwired: 1 in, 3 out]
          n463 = Match Pattern(string=w1036, regular expression=".lvclass") -> (before substring=w1031:string)  [unwired: 1 in, 3 out]
          n464 = Greater Or Equal To 0?(x=w1037) -> (x >= 0?=w1030:bool)
        }
        n465 = Close Reference(reference=w1021, error in (no error)=w1020) -> (error out=w1019:errorcluster)
      }
      frame Error {
        n466 = call <vilib>:"Clear Errors.vi"("error in (no error)"=w1042) -> ("error out"=w1041:errorcluster)  [unwired: 5 in, 1 out]
      }
    }
    n467 = Close Reference(reference=w1012, error in (no error)=w1009) -> (error out=w1006:errorcluster)
    n468 = Close Reference(reference=w1013, error in (no error)=w1006) -> (error out=w1005:errorcluster)
    n469 = Empty Array?(array=w1017) -> (empty?=w1004:bool)
    n470 = Not(x=w1004) -> (.not. x?=w1016:bool)
    n471 = call <vilib>:"Clear Errors.vi"("error in (no error)"=w1005) -> ("error out"=w1002:errorcluster)  [unwired: 5 in, 1 out]
    n472 = property on="RootClass" class="Ring (strict)"(error in=w1002, "Strings []"=w1017, "Visible"=w1016, "Value"=0) -> (error out=w1003:errorcluster)  [unwired: 1 in, 1 out]
    n473 = property on="OpClnUI" class="Bool"(error in=w1003, "Visible"=w1016) -> (error out=w999:errorcluster)  [unwired: 1 in, 1 out]
  }
  n474 = Unregister For Events(event registration refnum=w13, error in=w15) -> (error out=w14:errorcluster)
  n475 = Unregister For Events(event registration refnum=w17, error in=w18) -> (error out=w16:errorcluster)
  n476 = Merge Errors(w16, w14, w5) -> (w20:errorcluster)
  n477 = call <vilib>:"G#Debugger_Close.vi"("refs"=w21, "error in (no error)"=w20) -> ("error out"=w7:errorcluster)  [unwired: 17 in]
  n478 = case shown="No Error" w7 {
    selector: w7 -> [w1043 w1045]
    tunnel: [w1043 _] -> w8
    frame No Error {
    }
    frame Error {
      n479 = Unbundle By Name(w1045) -> ("source"=w1044:string)
      n480 = One Button Dialog(message=w1044) -> ()  [unwired: 1 in, 1 out]
    }
  }
  n481 = invoke class="VI" method="FP.Close"(error in=w8) -> ()  [unwired: 2 in, 3 out]
